vi "main 0.9.1.vi"() -> ()   [LabVIEW 2020]
uses:
  subvi/Newport ESP301/Newport ESP301.lvlib
  subvi/sp_manip.llb/sp_manip_lib.lvlib
  subvi/sp_manip.llb/tcp_gateway.lvlib
  subvi/PHOIBOS/DEFINITIONS/DEF_dev_type.ctl
  subvi/PHOIBOS/DEFINITIONS/DEF_dev_state.ctl
  <vilib>/Utility/file.llb/Write Delimited Spreadsheet (DBL).vi
  <vilib>/Utility/file.llb/Read Delimited Spreadsheet (string).vi
  <vilib>/Analysis/NI_AALBase.lvlib
  <vilib>/Analysis/1siggen.llb/Ramp Pattern by Samples.vi
panel:
  out "Waveform Chart":dbl(graph)
  out "G2 X":cluster{dbl[], "Ramp Pattern":dbl[]}(graph)={array[344 elements], "Ramp Pattern"=[5593.0, 5541.0, 5578.0, 5573.0, 5542.0, 5582.0, 5523.0, 5570.0, 5578.0, 5560.0, 5581.0, 5542.0, 5577.0, 5517.0, 5599.0, 5558.0, 5549.0, 5571.0, 5527.0, 5574.0, 5565.0, 5561.0, 5570.0, 5531.0, 5576.0, 5531.0, 5576.0, 5554.0, 5523.0, 5573.0, 5536.0, 5555.0, 5539.0, 5549.0, 5543.0, 5541.0, 5581.0, 5523.0, 5548.0, 5528.0, 5558.0, 5565.0, 5537.0, 5556.0, 5521.0, 5538.0, 5549.0, 5532.0, 5562.0, 5512.0, 5555.0, 5549.0, 5536.0, 5542.0, 5511.0, 5567.0, 5526.0, 5549.0, 5545.0, 5543.0, 5562.0, 5518.0, 5561.0, 5490.0, 5542.0, 5522.0, 5529.0, 5542.0, 5521.0, 5556.0, 5511.0, 5541.0, 5534.0, 5512.0, 5569.0, 5525.0, 5547.0, 5507.0, 5533.0, 5533.0, 5501.0, 5555.0, 5497.0, 5517.0, 5526.0, 5519.0, 5565.0, 5503.0, 5548.0, 5496.0, 5544.0, 5523.0, 5534.0, 5533.0, 5501.0, 5529.0, 5494.0, 5523.0, 5526.0, 5519.0, 5539.0, 5493.0, 5508.0, 5532.0, 5504.0, 5546.0, 5540.0, 5550.0, 5488.0, 5556.0, 5535.0, 5510.0, 5535.0, 5515.0, 5543.0, 5475.0, 5538.0, 5528.0, 5504.0, 5523.0, 5502.0, 5535.0, 5473.0, 5503.0, 5501.0, 5531.0, 5525.0, 5490.0, 5524.0, 5484.0, 5520.0, 5506.0, 5492.0, 5516.0, 5477.0, 5511.0, 5487.0, 5509.0, 5496.0, 5467.0, 5538.0, 5494.0, 5512.0, 5497.0, 5498.0, 5526.0, 5482.0, 5506.0, 5466.0, 5522.0, 5489.0, 5512.0, 5518.0, 5475.0, 5547.0, 5480.0, 5569.0, 5504.0, 5485.0, 5528.0, 5506.0, 5529.0, 5468.0, 5524.0, 5507.0, 5518.0, 5511.0, 5471.0, 5525.0, 5480.0, 5482.0, 5510.0, 5506.0, 5522.0, 5475.0, 5540.0, 5477.0, 5511.0, 5514.0, 5500.0, 5497.0, 5484.0, 5536.0, 5476.0, 5485.0, 5527.0, 5509.0, 5529.0, 5495.0, 5504.0, 5496.0, 5519.0, 5512.0, 5469.0, 5506.0, 5465.0, 5502.0, 5481.0, 5508.0, 5519.0, 5499.0, 5515.0, 5476.0, 5496.0, 5502.0, 5499.0, 5494.0, 5477.0, 5541.0, 5477.0, 5512.0, 5497.0, 5472.0, 5511.0, 5471.0, 5503.0, 5507.0, 5504.0, 5477.0, 5479.0, 5508.0, 5481.0, 5522.0, 5517.0, 5516.0, 5505.0, 5502.0, 5491.0, 5481.0, 5512.0, 5484.0, 5500.0, 5478.0, 5493.0, 5529.0, 5492.0, 5518.0, 5471.0, 5518.0, 5490.0, 5513.0, 5497.0, 5488.0, 5517.0, 5477.0, 5524.0, 5464.0, 5495.0, 5514.0, 5495.0, 5522.0, 5477.0, 5490.0, 5535.0, 5489.0, 5491.0, 5491.0, 5515.0, 5473.0, 5504.0, 5505.0, 5515.0, 5510.0, 5473.0, 5521.0, 5475.0, 5537.0, 5499.0, 5505.0, 5509.0, 5460.0, 5509.0, 5473.0, 5489.0, 5500.0, 5464.0, 5522.0, 5471.0, 5528.0, 5475.0, 5502.0, 5494.0, 5511.0, 5516.0, 5486.0, 5528.0, 5471.0, 5492.0, 5477.0, 5491.0, 5531.0, 5486.0, 5549.0, 5498.0, 5524.0, 5482.0, 5495.0, 5505.0, 5476.0, 5512.0, 5444.0, 5512.0, 5498.0, 5471.0, 5489.0, 5462.0, 5502.0, 5459.0, 5503.0, 5489.0, 5493.0, 5498.0, 5461.0, 5505.0, 5495.0, 5503.0, 5459.0, 5501.0, 5515.0, 5459.0, 5510.0, 5469.0, 5504.0, 5499.0, 5505.0, 5524.0, 5477.0, 5527.0, 5477.0, 5475.0, 5495.0, 5482.0, 5514.0, 5481.0, 5499.0, 5481.0, 5482.0, 5498.0, 5460.0, 5469.0, 5471.0, 5519.0, 5495.0, 5485.0]}
  in  "reset every n pics":bool
  in  "pics2avg":i32=50
  in  "abort acq.":bool
  out "G2 Y":cluster{dbl[], "Ramp Pattern":dbl[]}(graph)={[5738.0, 5692.0, 5562.0, 5630.0, 5633.0, 5616.0, 5523.0, 5622.0, 5406.0, 5598.0, 5416.0, 5403.0, 5579.0, 5325.0, 5504.0, 5402.0, 5538.0, 5568.0, 5460.0, 5494.0, 5367.0, 5597.0, 5434.0, 5448.0, 5339.0, 5434.0, 5460.0, 5482.0, 5646.0, 5720.0, 5704.0, 5628.0, 5672.0, 5511.0, 5420.0, 5539.0, 5543.0, 5421.0, 5486.0, 5508.0, 5537.0, 5586.0, 5460.0, 5547.0, 5433.0, 5488.0, 5552.0, 5538.0, 5528.0, 5482.0, 5406.0, 5458.0, 5644.0, 5485.0, 5443.0, 5485.0, 5385.0, 5413.0, 5472.0, 5571.0, 5640.0, 5602.0, 5462.0, 5477.0, 5408.0, 5396.0, 5445.0, 5638.0, 5383.0, 5571.0, 5372.0, 5519.0, 5426.0, 5462.0, 5481.0, 5626.0, 5326.0, 5458.0, 5471.0, 5366.0, 5394.0, 5363.0, 5551.0, 5596.0, 5452.0, 5470.0, 5600.0, 5533.0, 5573.0, 5544.0, 5671.0, 5595.0, 5423.0, 5550.0, 5557.0, 5416.0, 5404.0, 5478.0, 5448.0, 5512.0, 5505.0, 5575.0, 5434.0, 5436.0, 5600.0, 5487.0, 5607.0, 5463.0, 5606.0, 5540.0, 5521.0, 5581.0, 5472.0, 5555.0, 5576.0, 5612.0, 5529.0, 5473.0, 5454.0, 5455.0, 5500.0, 5650.0, 5451.0, 5445.0, 5423.0, 5376.0, 5389.0, 5491.0, 5536.0, 5525.0, 5440.0, 5707.0, 5414.0, 5532.0, 5400.0, 5668.0, 5706.0, 5515.0, 5431.0, 5400.0, 5439.0, 5471.0, 5627.0, 5691.0, 5569.0, 5718.0, 5614.0, 5523.0, 5436.0, 5432.0, 5419.0, 5516.0, 5469.0, 5467.0, 5530.0, 5598.0, 5501.0, 5476.0, 5457.0, 5460.0, 5606.0, 5456.0, 5429.0, 5586.0, 5504.0, 5546.0, 5516.0, 5466.0, 5650.0, 5593.0, 5605.0, 5515.0, 5414.0, 5623.0, 5581.0, 5651.0, 5574.0, 5519.0, 5672.0, 5621.0, 5496.0, 5382.0, 5496.0, 5620.0, 5542.0, 5422.0, 5492.0, 5515.0, 5549.0, 5402.0, 5472.0, 5547.0, 5515.0, 5641.0, 5451.0, 5667.0, 5622.0, 5511.0, 5506.0, 5608.0, 5647.0, 5584.0, 5714.0, 5490.0, 5534.0, 5463.0, 5566.0, 5573.0, 5570.0, 5582.0, 5613.0, 5504.0, 5550.0, 5594.0, 5576.0, 5677.0, 5675.0, 5681.0, 5681.0, 5434.0, 5434.0, 5405.0, 5473.0, 5522.0, 5427.0, 5533.0, 5582.0, 5427.0, 5529.0, 5548.0, 5341.0, 5521.0, 5539.0, 5435.0, 5457.0, 5511.0, 5406.0, 5412.0, 5620.0, 5609.0, 5609.0, 5469.0, 5577.0, 5661.0, 5673.0, 5518.0, 5463.0, 5562.0, 5723.0, 5719.0, 5487.0, 5485.0, 5683.0, 5501.0, 5604.0, 5328.0], "Ramp Pattern"=[0.0, 1.003921568627451, 2.007843137254902, 3.011764705882353, 4.015686274509804, 5.019607843137255, 6.023529411764706, 7.027450980392157, 8.031372549019608, 9.035294117647059, 10.03921568627451, 11.04313725490196, 12.047058823529412, 13.050980392156863, 14.054901960784314, 15.058823529411764, 16.062745098039215, 17.066666666666666, 18.070588235294117, 19.07450980392157, 20.07843137254902, 21.08235294117647, 22.08627450980392, 23.090196078431372, 24.094117647058823, 25.098039215686274, 26.101960784313725, 27.105882352941176, 28.109803921568627, 29.113725490196078, 30.11764705882353, 31.12156862745098, 32.12549019607843, 33.129411764705885, 34.13333333333333, 35.13725490196079, 36.141176470588235, 37.14509803921569, 38.14901960784314, 39.15294117647059, 40.15686274509804, 41.16078431372549, 42.16470588235294, 43.168627450980395, 44.17254901960784, 45.1764705882353, 46.180392156862744, 47.1843137254902, 48.188235294117646, 49.1921568627451, 50.19607843137255, 51.2, 52.20392156862745, 53.207843137254905, 54.21176470588235, 55.21568627450981, 56.219607843137254, 57.22352941176471, 58.227450980392156, 59.23137254901961, 60.23529411764706, 61.23921568627451, 62.24313725490196, 63.247058823529414, 64.25098039215686, 65.25490196078431, 66.25882352941177, 67.26274509803922, 68.26666666666667, 69.27058823529411, 70.27450980392157, 71.27843137254902, 72.28235294117647, 73.28627450980392, 74.29019607843138, 75.29411764705883, 76.29803921568627, 77.30196078431372, 78.30588235294118, 79.30980392156863, 80.31372549019608, 81.31764705882352, 82.32156862745099, 83.32549019607843, 84.32941176470588, 85.33333333333333, 86.33725490196079, 87.34117647058824, 88.34509803921569, 89.34901960784313, 90.3529411764706, 91.35686274509804, 92.36078431372549, 93.36470588235294, 94.3686274509804, 95.37254901960785, 96.37647058823529, 97.38039215686274, 98.3843137254902, 99.38823529411765, 100.3921568627451, 101.39607843137254, 102.4, 103.40392156862745, 104.4078431372549, 105.41176470588235, 106.41568627450981, 107.41960784313726, 108.4235294117647, 109.42745098039215, 110.43137254901961, 111.43529411764706, 112.43921568627451, 113.44313725490196, 114.44705882352942, 115.45098039215686, 116.45490196078431, 117.45882352941176, 118.46274509803922, 119.46666666666667, 120.47058823529412, 121.47450980392156, 122.47843137254903, 123.48235294117647, 124.48627450980392, 125.49019607843137, 126.49411764705883, 127.49803921568628, 128.50196078431372, 129.50588235294117, 130.50980392156862, 131.51372549019607, 132.51764705882354, 133.521568627451, 134.52549019607844, 135.52941176470588, 136.53333333333333, 137.53725490196078, 138.54117647058823, 139.54509803921567, 140.54901960784315, 141.5529411764706, 142.55686274509804, 143.5607843137255, 144.56470588235294, 145.5686274509804, 146.57254901960783, 147.57647058823528, 148.58039215686276, 149.5843137254902, 150.58823529411765, 151.5921568627451, 152.59607843137255, 153.6, 154.60392156862744, 155.6078431372549, 156.61176470588236, 157.6156862745098, 158.61960784313726, 159.6235294117647, 160.62745098039215, 161.6313725490196, 162.63529411764705, 163.6392156862745, 164.64313725490197, 165.64705882352942, 166.65098039215687, 167.65490196078431, 168.65882352941176, 169.6627450980392, 170.66666666666666, 171.6705882352941, 172.67450980392158, 173.67843137254903, 174.68235294117648, 175.68627450980392, 176.69019607843137, 177.69411764705882, 178.69803921568626, 179.7019607843137, 180.7058823529412, 181.70980392156864, 182.71372549019608, 183.71764705882353, 184.72156862745098, 185.72549019607843, 186.72941176470587, 187.73333333333332, 188.7372549019608, 189.74117647058824, 190.7450980392157, 191.74901960784314, 192.75294117647059, 193.75686274509803, 194.76078431372548, 195.76470588235293, 196.7686274509804, 197.77254901960785, 198.7764705882353, 199.78039215686275, 200.7843137254902, 201.78823529411764, 202.7921568627451, 203.79607843137254, 204.8, 205.80392156862746, 206.8078431372549, 207.81176470588235, 208.8156862745098, 209.81960784313725, 210.8235294117647, 211.82745098039214, 212.83137254901962, 213.83529411764707, 214.8392156862745, 215.84313725490196, 216.8470588235294, 217.85098039215686, 218.8549019607843, 219.85882352941175, 220.86274509803923, 221.86666666666667, 222.87058823529412, 223.87450980392157, 224.87843137254902, 225.88235294117646, 226.8862745098039, 227.89019607843136, 228.89411764705883, 229.89803921568628, 230.90196078431373, 231.90588235294118, 232.90980392156862, 233.91372549019607, 234.91764705882352, 235.92156862745097, 236.92549019607844, 237.9294117647059, 238.93333333333334, 239.93725490196078, 240.94117647058823, 241.94509803921568, 242.94901960784313, 243.95294117647057, 244.95686274509805, 245.9607843137255, 246.96470588235294, 247.9686274509804, 248.97254901960784, 249.9764705882353, 250.98039215686273, 251.98431372549018, 252.98823529411766, 253.9921568627451, 254.99607843137255, 256.0]}
  out "ETA":timestamp=timestamp(3543843884.995538 s since 1904-01-01) format="%<%H:%M:%S>T"
  out "acq. imgs":i32=30
  out "snap_prog":dbl(slide)=1.0 scale=0.0..1.0
  in  "BasePath":path=path "Z:/PESdata"
  in  "cam_liveavg":bool caption="live average"
  out "cam_fps":dbl=20.079713544692744 caption="FPS" format="%.1g"
  out "sideimg":dbl[][](graph)
  in  "RunNumber":u16=77
  out "sum":dbl=4126991.0 format="%#.2g"
  out "max":dbl=54.0
  out "mainimg":dbl[][](graph)
  out "ESP_con?":bool=TRUE caption="ESP301"
  out "phoib_con?":bool caption="PHOIBOS"
  out "manip_con?":bool caption="manipulator"
  out "cam_con?":bool caption="camera"
  in  "main_close":bool
  in  "Tab Control":T1(tab)
  in  "manip_deltas":dbl[](array[numeric])=[0.0, 0.0, 0.0, 0.0, 10.0, 0.0] caption="delta" format="%#.5g"
  in  "aq.mode":enum32{"Radio Selection 1", "Radio Selection 2"}(radio)=enum."Radio Selection 2"
  in  "dark avg":i32=100
  in  "averages":i32=30 caption="N"
  in  "ESP_delta":dbl caption="relative [mm]"
  in  "ESP_-":bool
  in  "ESP_+":bool
  in  "ESP_go":bool
  in  "ESP_dest_t":dbl=250.17307139859977 caption="[fs]"
  in  "ESP_dest":dbl=31.304 caption="[mm]"
  in  "ESP_set_t0":bool
  in  "phoib_I_6s":dbl=3200.0
  in  "phoib_I_5s":dbl=1650.0
  in  "phoib_I_4s":dbl=4.558
  in  "phoib_I_3s":dbl=-7.0
  in  "phoib_I_2s":dbl=20.0
  in  "phoib_I_1s":dbl=22.0
  in  "phoib_standby":bool
  in  "phoib_set":bool
  out "phoib_I_6":dbl caption="Screen Voltage"
  out "phoib_I_5":dbl caption="Detctor Voltage"
  out "phoib_I_4":dbl caption="Work Function"
  out "phoib_I_3":dbl caption="Coil Current"
  out "phoib_I_2":dbl caption="Pass Energy"
  out "phoib_I_1":dbl caption="Kinetic Energy"
  out "Saved Positions":string[][](table)=[["ertwertwert", "-2.299945", "-2.030214", "38.900024", "50.000762", "0.000887", "-97.998082"], ["uztgugt", "-14.999451", "-13.638894", "442.380066", "13.998380", "-1.893758", "-76.305838"], ["asdf", "-14.999451", "-13.638894", "442.380066", "13.998380", "-1.893758", "-76.305838"], ["test3", "-14.999451", "-13.638894", "441.380066", "13.998380", "-1.893758", "-76.305838"]]
  in  "Save Pos":bool
  in  "Load":bool
  in  "Delete":bool
  in  "ManipRel +":bool
  in  "ManipRel -":bool
  in  "Move Abs":bool
  in  "stop manip":bool
  in  "dest":dbl[](array[numeric])=[-2.6172862113166087, -0.009888298846365134, 68.5008544921875, -46.36280498847848, 1.1073518432055398, -218.56360350415366] caption="destination" format="%#.5g"
  out "axis":string[](array[string])=["x", "y", "z", "polar", "tilt", "azimut"]
  out "pos":dbl[](array[numeric])=[-2.6172862113166087, -0.009888298846365134, 68.5008544921875, -46.363686276590336, 11.108982061941884, -218.56360350415366] caption="position" format="%.5f"
  in  "Mode":T2(ring)=enum."WideAngleMode"
  in  "VoltageRange":enum16{"3.5kV", "1.5kV", "400V", "100V", "10V"}(ring)=enum."400V"
  out "ESP_pos":dbl=31.4539 caption="Position"
  out "ESP_delay":dbl=1000.0251574040756 caption="Delay"
  out "ESP_t0":dbl=31.304 caption="Time Zero @"
  out "phoib_I_7":dbl caption="Conversion Voltage"
  in  "phoib_I_7s":dbl=-16.0
  in  "phoib_I_8s":dbl=0.0039
  in  "phoib_I_9s":dbl=0.0039
  out "phoib_I_8":dbl caption="FD1"
  out "phoib_I_9":dbl caption="FD2"
  in  "gain":bool
  in  "exposure [ms]":u32=1
  in  "binning":u16(ring)=2 items=["X 1", "X 2", "X 4", "X 8"]
  in  "cam_dark?":bool caption="subtract dark?"
  in  "cam_dark":bool
  in  "cam_saveimg":bool
  in  "e-size":u8
  in  "lower threshold":i32=-100
  in  "count?":bool
  in  "ROI Left":i32=1
  in  "ROI Right":i32=43
  in  "ROI Top":i32=1
  in  "ROI Bottom":i32=33
  out "moving?":bool[](array[boolean])
  out "del_ETA":timestamp=timestamp(3543843871.185777 s since 1904-01-01) format="%<%H:%M:%S>T"
  out "time / step":dbl=2.792118032773336
  out "duration [HH:MM:SS]":dbl=55.62603882380894 format="%<%H:%M:%S>t"
  out "disk [MB]":dbl=11.613000000000001
  out "RAM [MB]":dbl=2.765
  out "total steps":dbl=20.0
  out "delaypoints":dbl=5.0
  in  "generate delay table":bool
  in  "load delay table":bool
  in  "delay table [fs]":string[][](table)=[["-1000.000000"], ["-500.000000"], ["0.000000"], ["500.000000"], ["1000.000000"]]
  in  "delscan_iters":u32=4 caption="iterations"
  out "scangraph":cluster{"delaypoints":dbl[], dbl[]}(graph)={"delaypoints"=[-1000.0, -500.0, 0.0, 500.0, 1000.0], [56872639.0, 56944859.59999999, 56835838.7999999, 56879783.599999934, 56864774.39999998]}
  in  "delscan_abort":bool
  out "delscan_progress":u32(slide)=5 scale=0.0..5.0
  in  "delscan_go":bool
  out "delscan_pos":dbl=31.453896228999998 caption="stage pos [mm]"
  in  "delscan_end":dbl=1000.0 caption="end [fs]"
  in  "delscan_stepsize":dbl=500.0 caption="stepsize [fs]"
  in  "delscan_start":dbl=-1000.0 caption="start [fs]"
  out "iteration":i32=5
  in  "delscan_finishIteration":bool
  in  "manip_scan_steps":u32=3
  in  "Optimize":bool
  in  "manip_scan_delta":dbl[](array[numeric])=[0.0, 0.0, 0.0, 0.0, 1.0, 0.0] caption="delta" format="%#.5g"
  out "delscan_progress 2":u32(slide)=2 scale=0.0..3.0
  in  "abort":bool
  in  "manip_init":bool
  in  "manip_release":bool
  in  "phoib_init":bool
  in  "phoib_release":bool
  in  "ESP_init":bool
  in  "ESP_release":bool
  in  "ESP301 VISA":refnum<visa-resource-name>="COM8"
  in  "board number":i32
  in  "cam_init":bool
  in  "cam_release":bool
  out "cam_error":errorcluster
  out "phoib_error":errorcluster
  out "state":T3 items=["Off"=-1, "Standby"=0, "On"=1]
  in  "ESP Axis":i32=1 min=1 max=3
  out "error out":errorcluster
  out "error out 2":errorcluster={"status"=TRUE, "code"=1, "source"="TCP Write in sp_manip_lib.lvlib:sp_manip_disconnect.vi->main 0.9.1.vi"}
  # "camera"
  # "analyzer"
  # "manipulator"
  # "aquisition"
  # "delay stage"
  # "Position"
  # "Destination"
  # "X\nY\nZ\npolar\ntilt\nazimut"
  # "camera"
  # "phoibos"
  # "ESP301"
  # "manipulator"
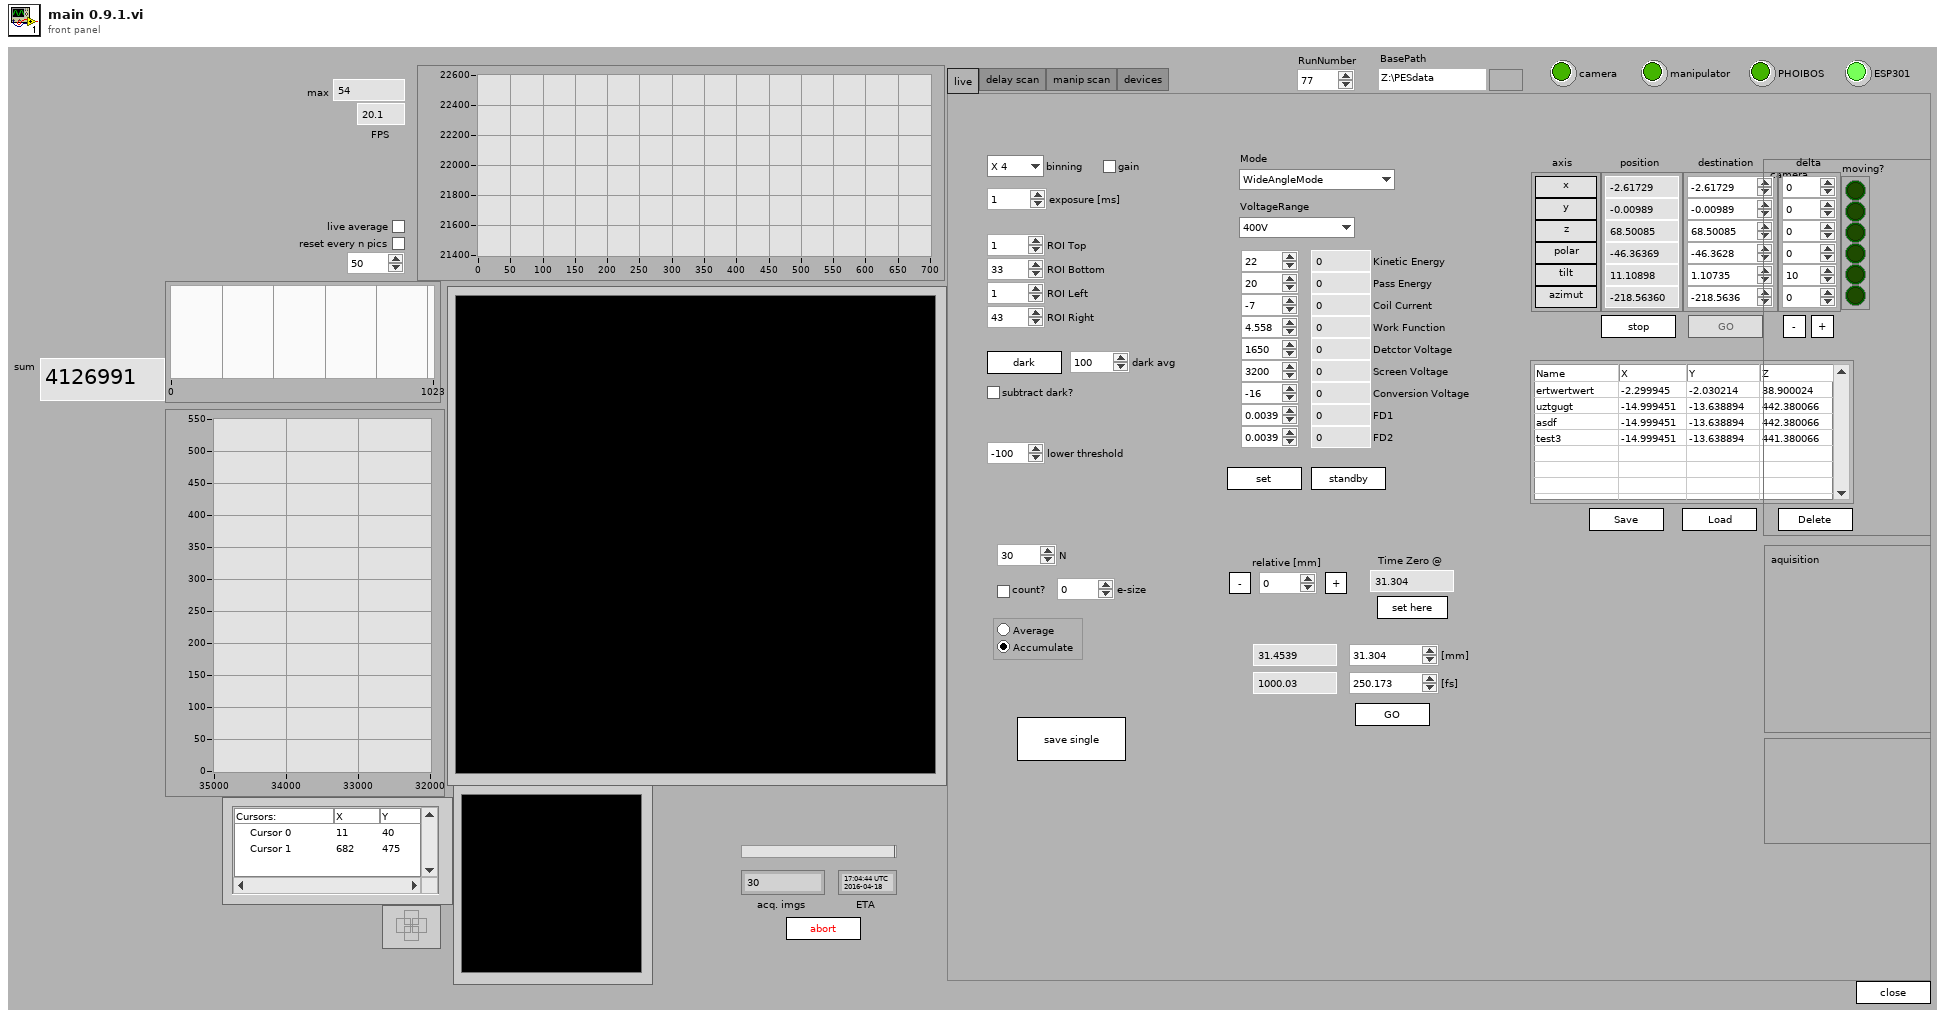
[diagram p1: front panel]
types:
  T1 = enum32{"live", "delay scan", "manip scan", "devices"}
  T2 = enum16{"HighMagnification", "MediumMagnification", "LowMagnification", "HighAngularDispersion", "MediumAngularDispersion", "LowAngularDispersion", "WideAngleMode", "LargeArea", "MediumArea", "SmallArea", "HighMagnification2", "SmallArea2", "ImagingMode"}
  T3 = typedef "DEF_dev_state.ctl" = i32
  T4 = typedef "LVCursorListTypeDef.ctl" = cluster{"Name":string, "Color":u32, "Style":u8, "Point Style":u8, "Name Visible":bool, "Allow Drag":bool, "Cursor Mode":u32, "Plot":i32, "Index":i32, "Position":cluster{"X":dbl, "Y":dbl}, "X Scale":u32, "Y Scale":u32, "Watch Plots":i32[], "Watch All Plots":bool, "Plot Area":i32, "Label Offset":cluster{"X":dbl, "Y":dbl}}[]
  T5 = cluster{"Camera type":u32, "Operating mode\nHP & QE / HS & DiCam Pro ":u32, "Frame trigger \n(High Performance and QE only)":u16, "Sequence trigger":u16, "Low Light\n(QE only)":bool, "Gain":bool, "Horzontal\nbinning":u16, "Vertical\nbinning ":u16, "ROI Left":i32, "ROI Right":i32, "ROI Top":i32, "ROI Bottom":i32}
  T6 = cluster{"Name":string, "Color":u32, "Style":u8, "Point Style":u8, "Name Visible":bool, "Allow Drag":bool, "Cursor Mode":u32, "Plot":i32, "Index":i32, "Position":cluster{"X":dbl, "Y":dbl}, "X Scale":u32, "Y Scale":u32, "Watch Plots":i32[], "Watch All Plots":bool, "Plot Area":i32, "Label Offset":cluster{"X":dbl, "Y":dbl}}
  T7 = cluster{"Axis_Name":string, "Axis_Type":string, "Axis_Position":dbl, "continous":bool, "moving":bool}[]
  T8 = typedef "DEF_dev_type.ctl" = enum32{"devA (analyzer)", "devD (detector)"}
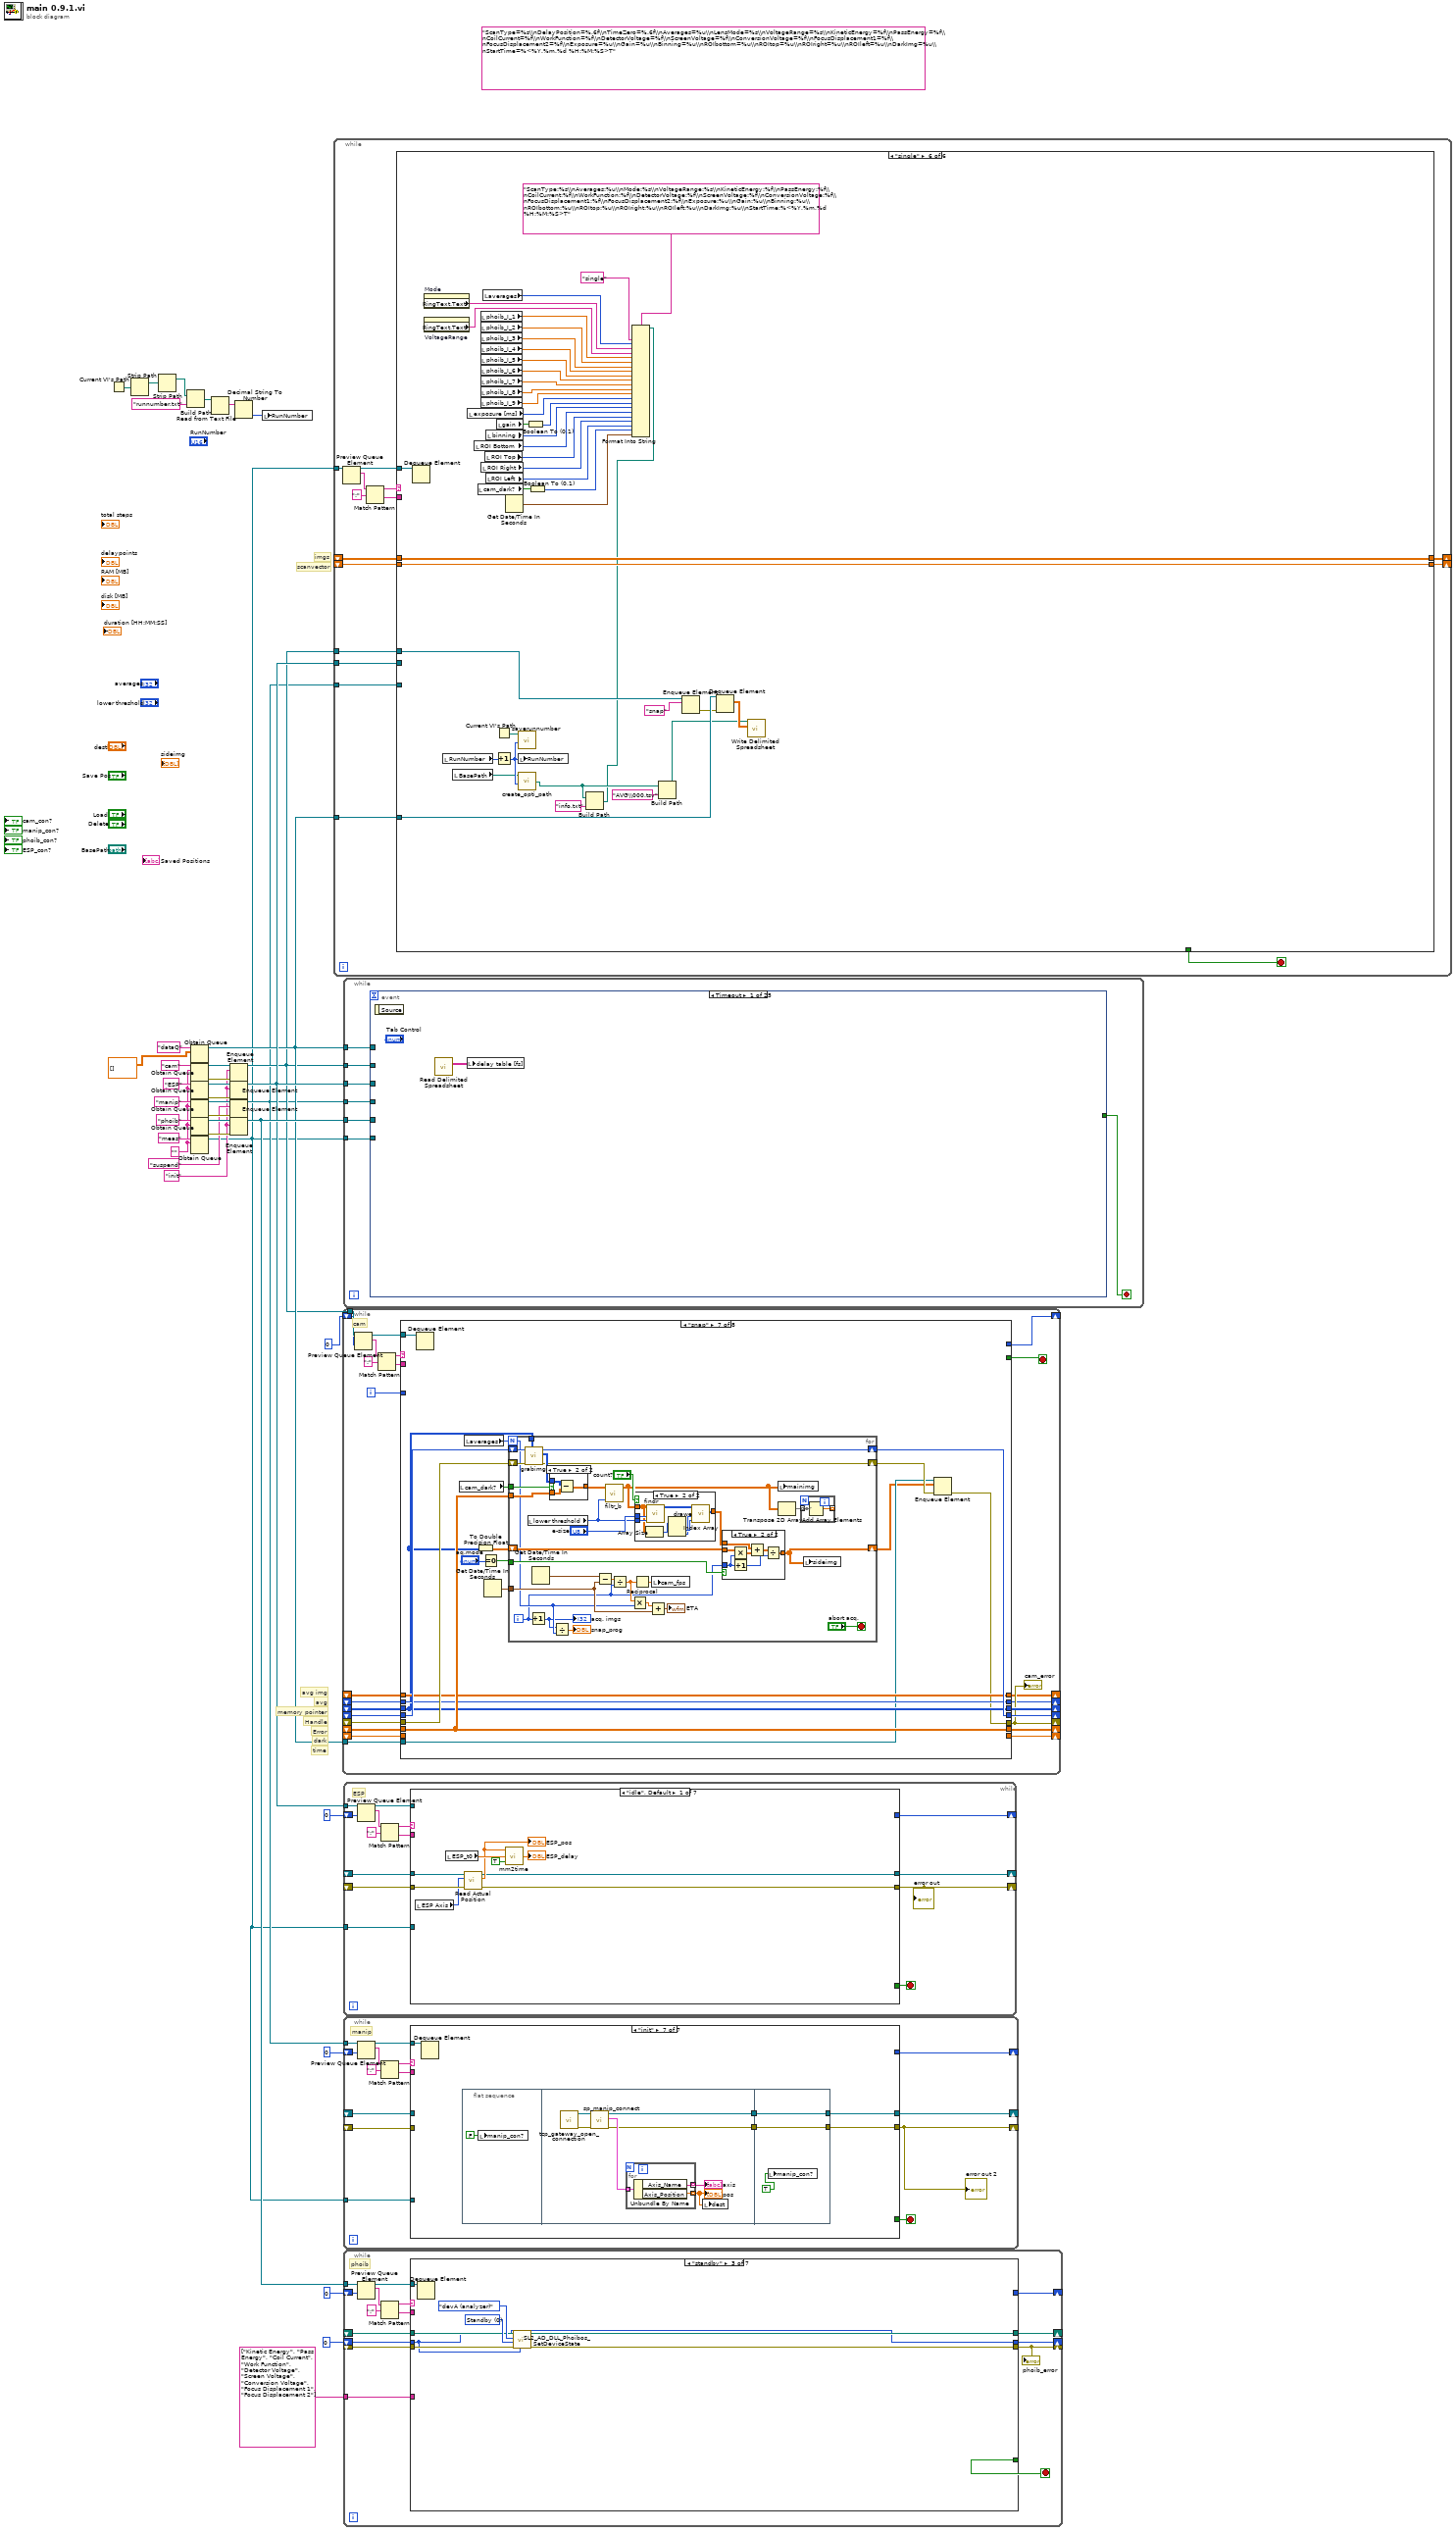
[diagram p0: block diagram]
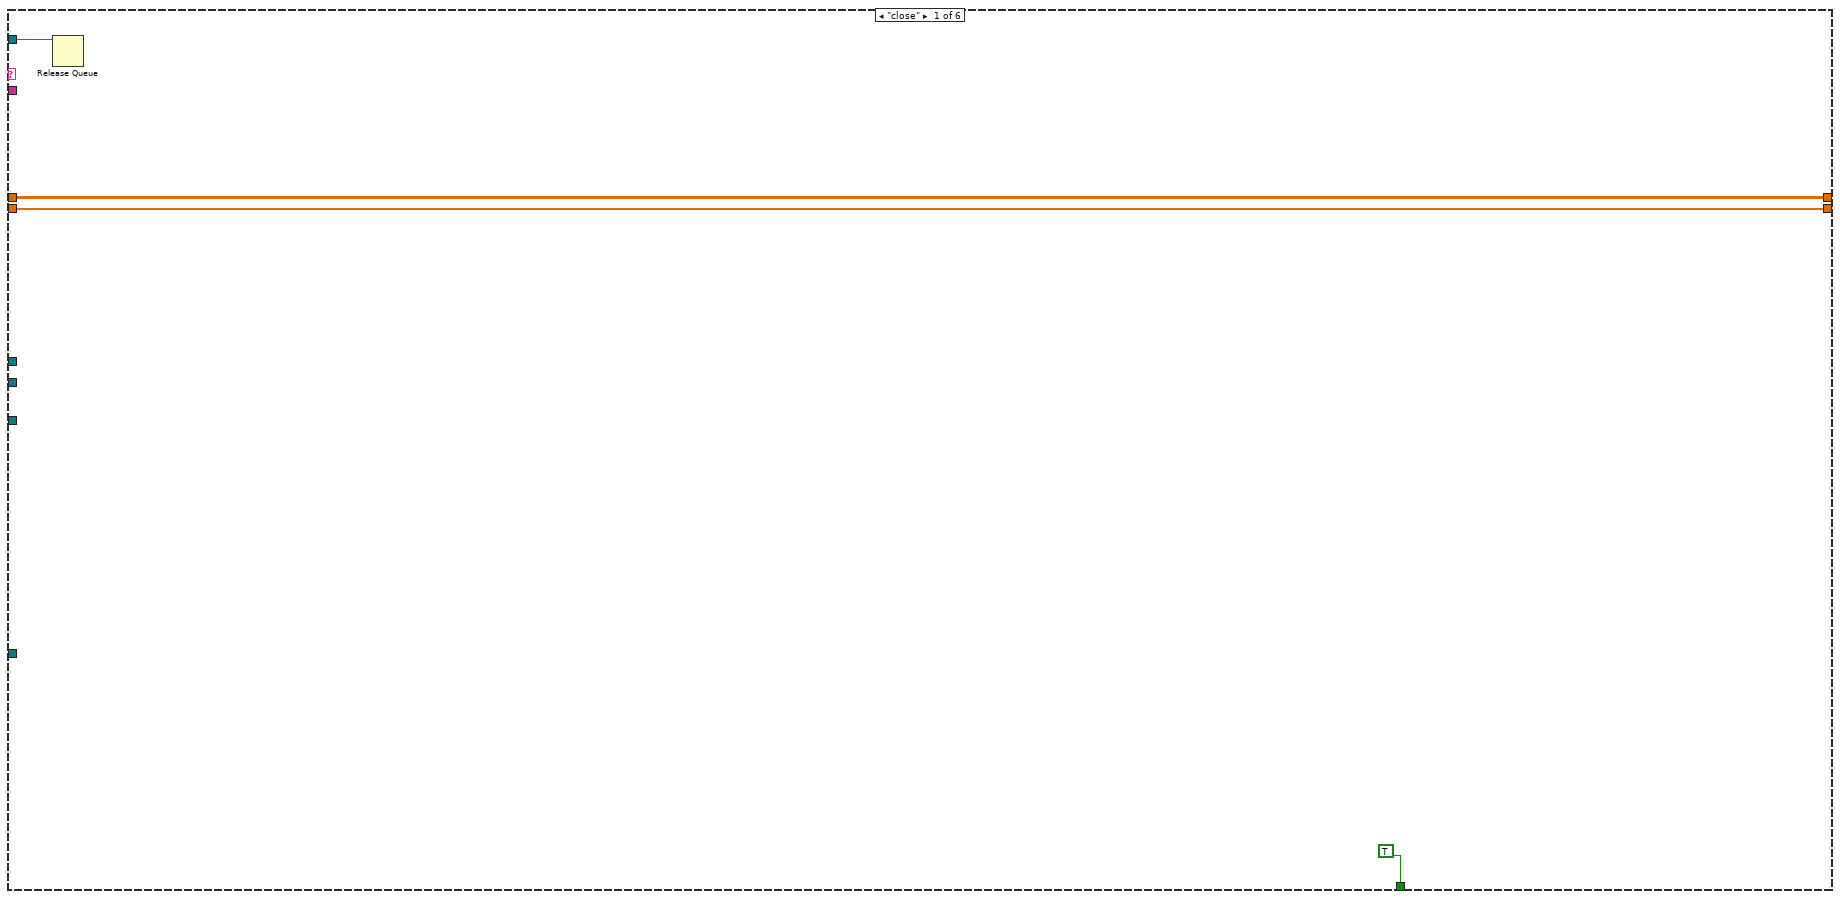
[diagram p2: hidden frame]
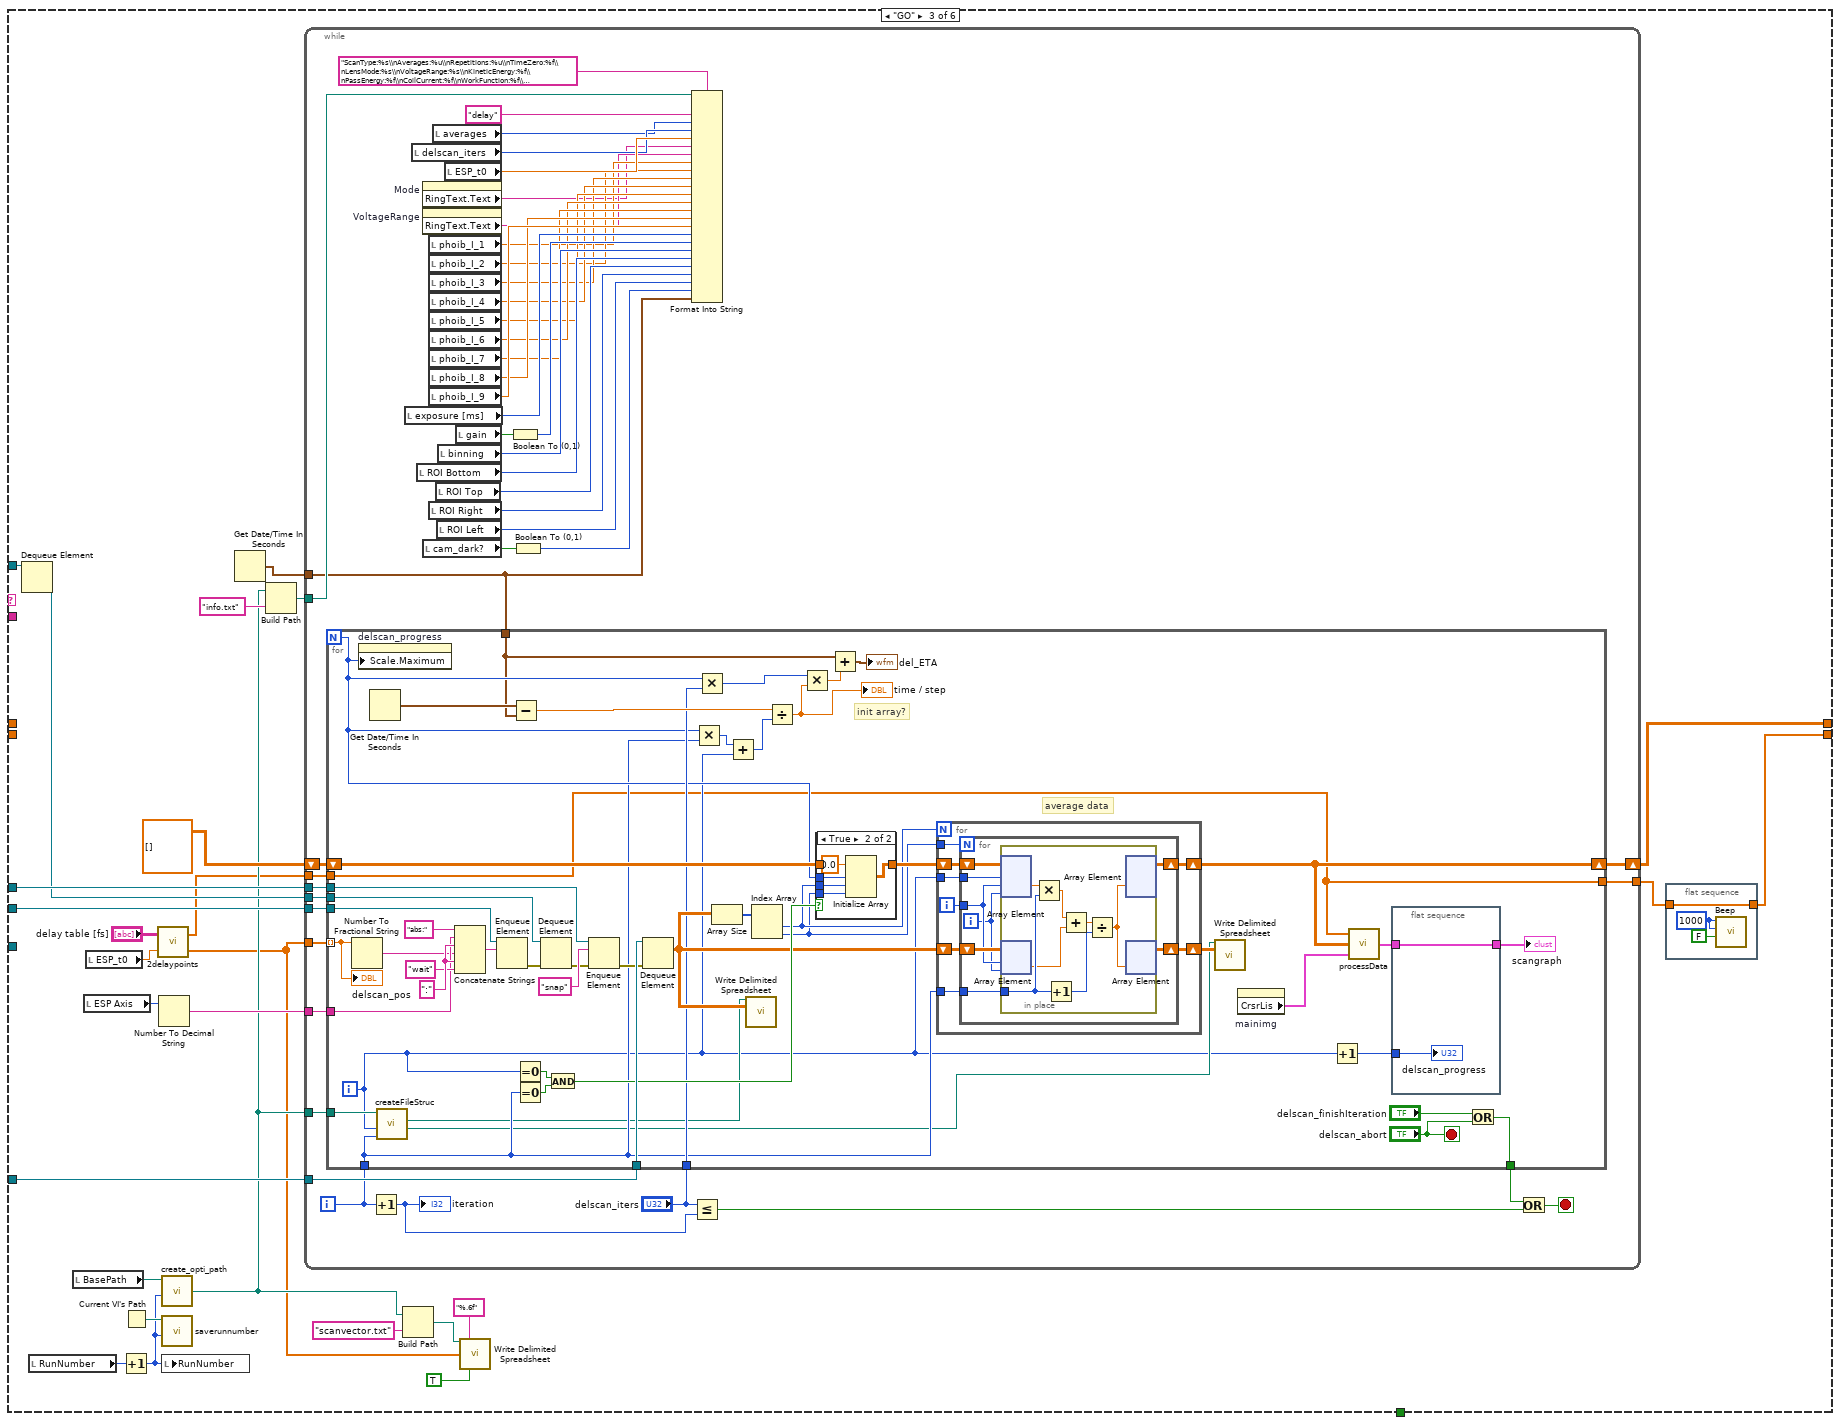
[diagram p4: hidden frame]
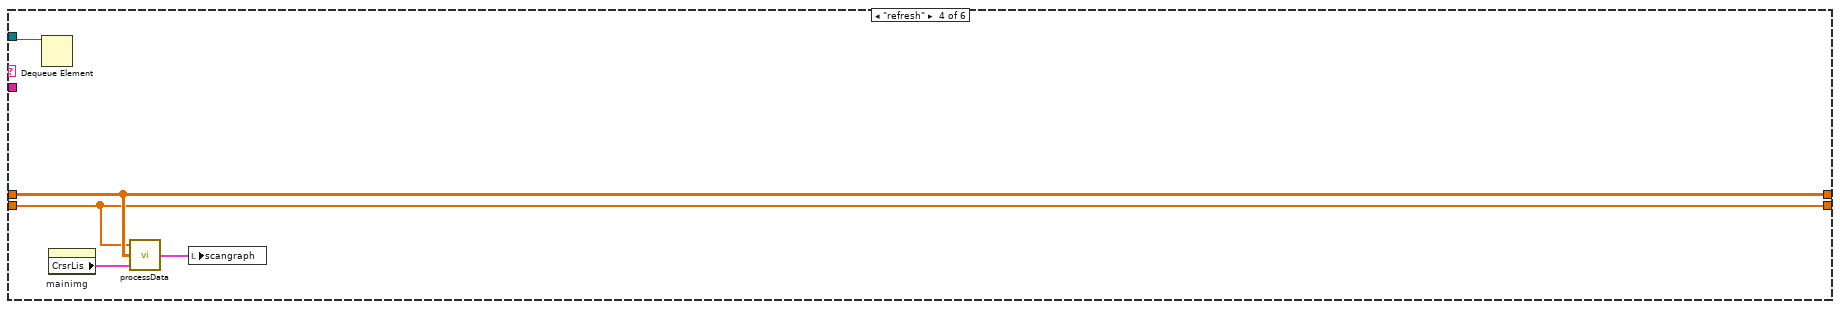
[diagram p6: hidden frame]
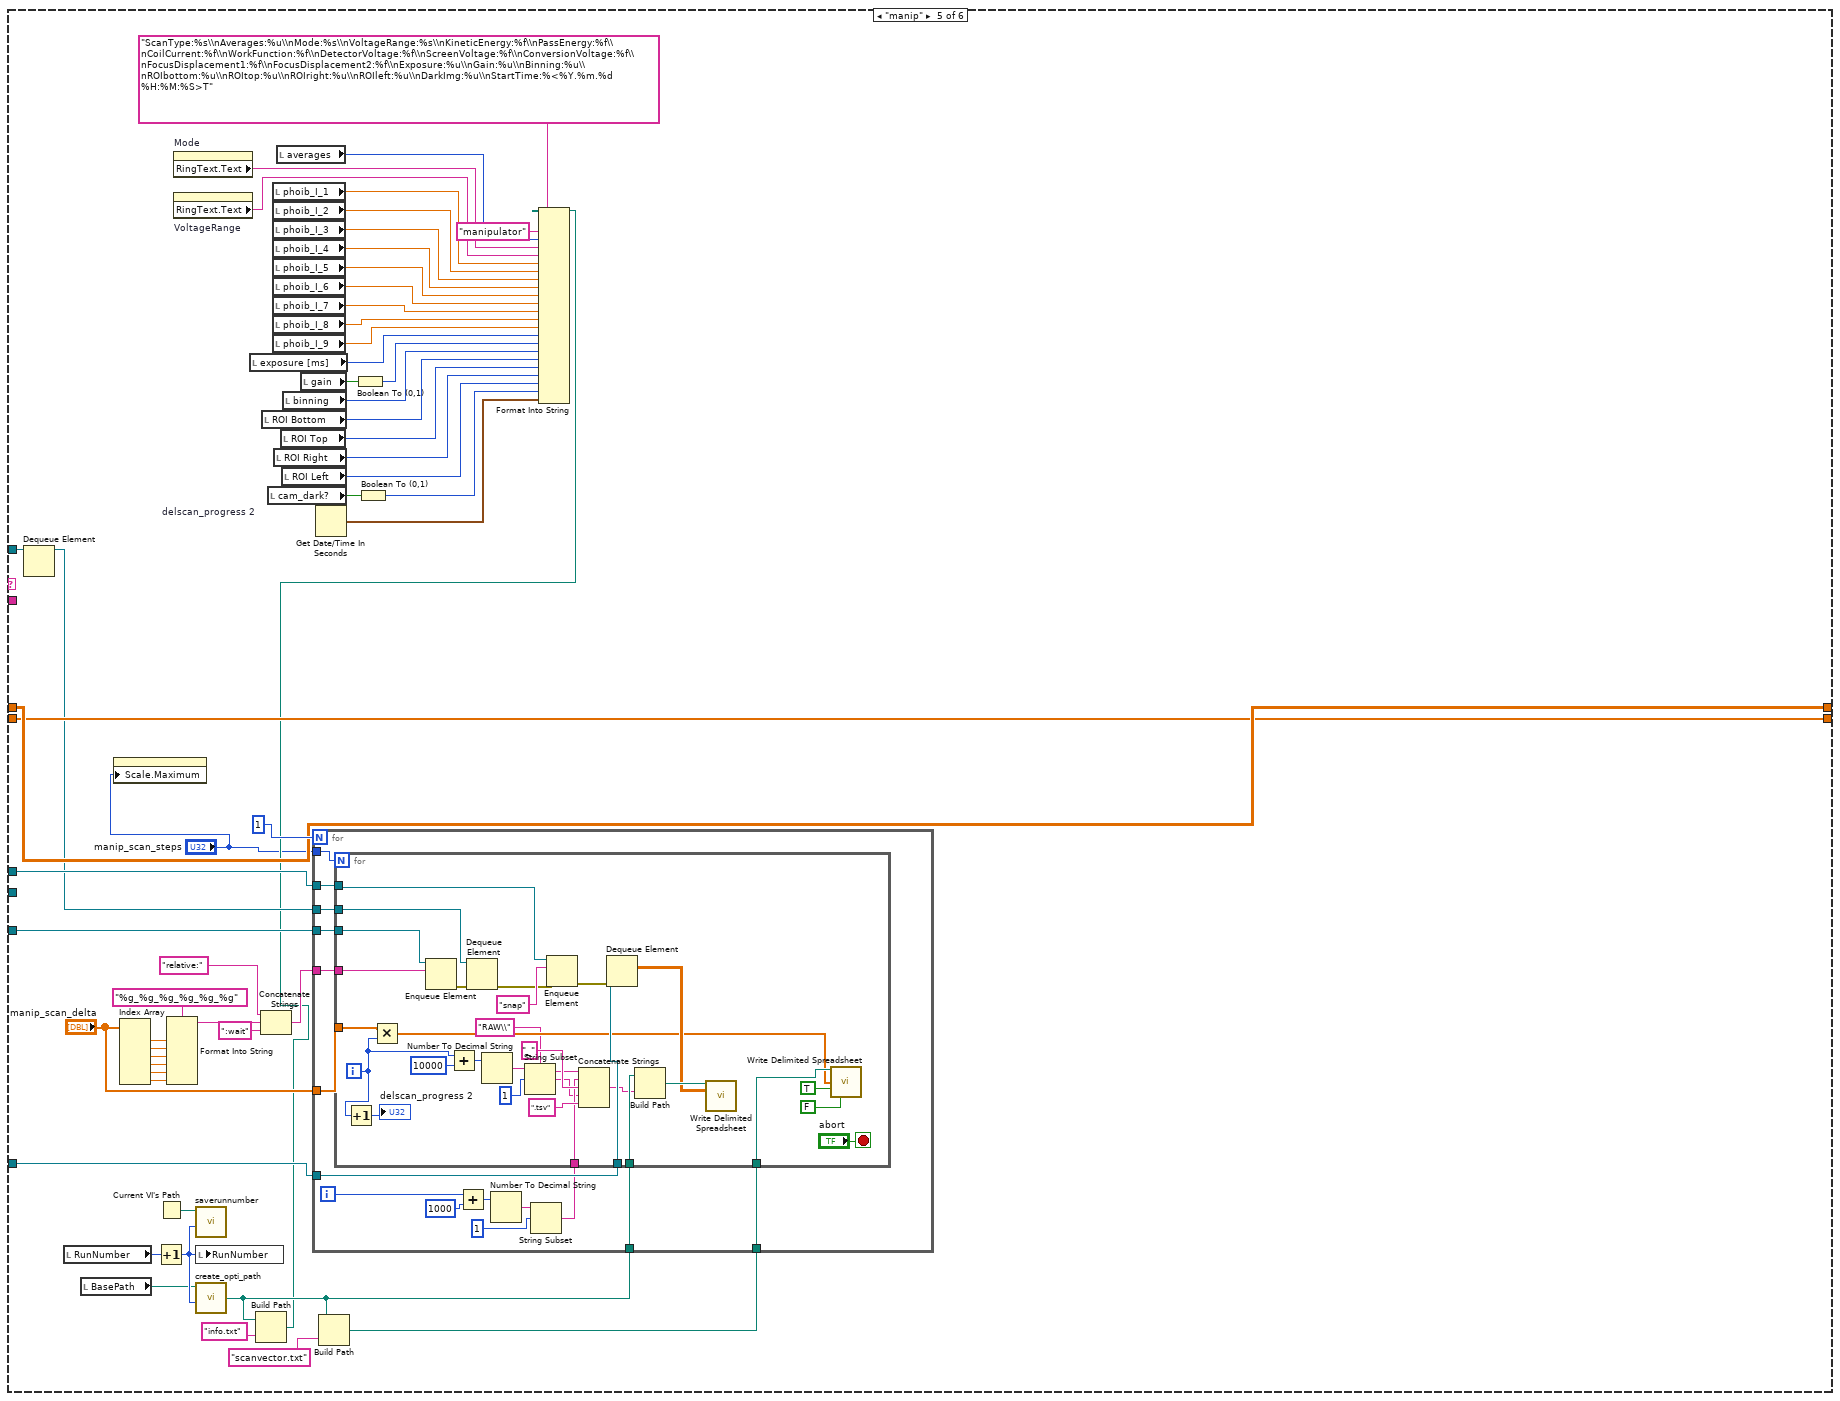
[diagram p7: hidden frame]
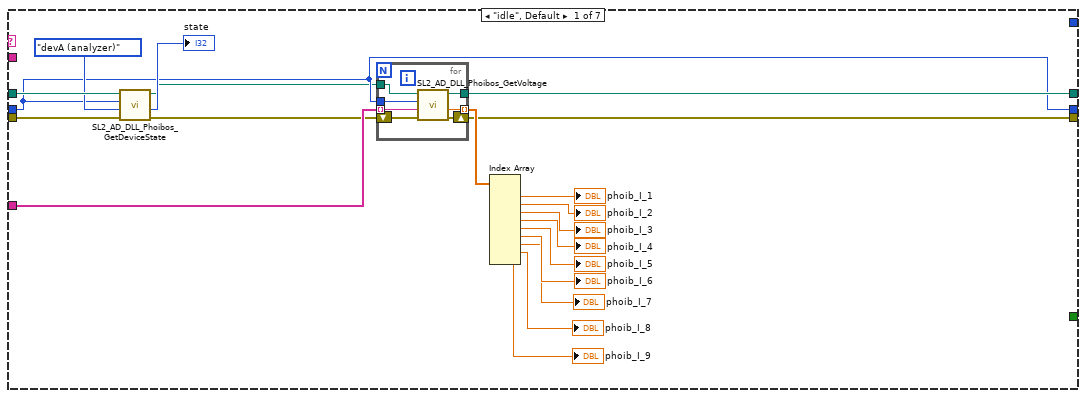
[diagram p8: hidden frame]
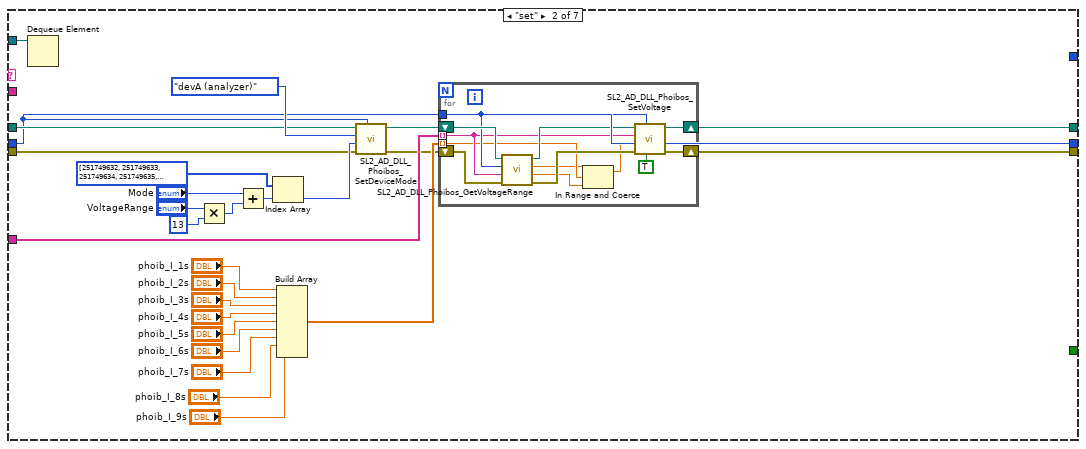
[diagram p9: hidden frame]
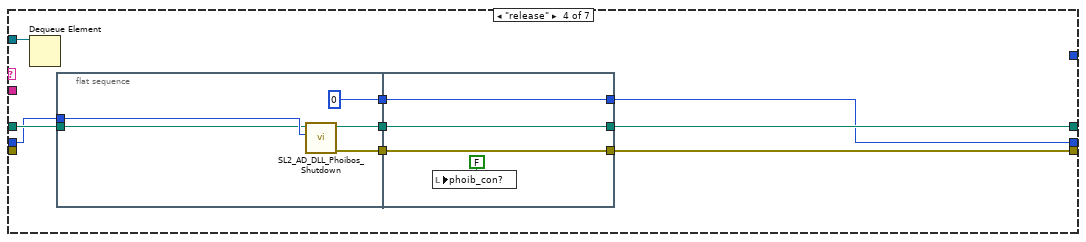
[diagram p10: hidden frame]
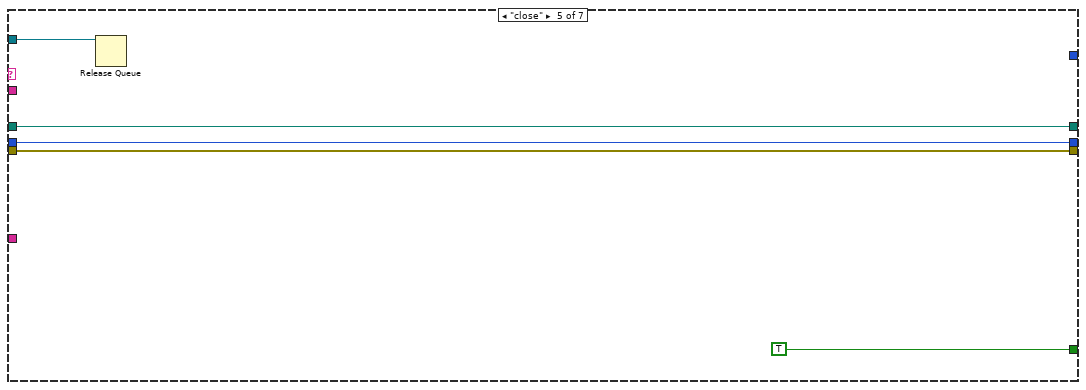
[diagram p11: hidden frame]
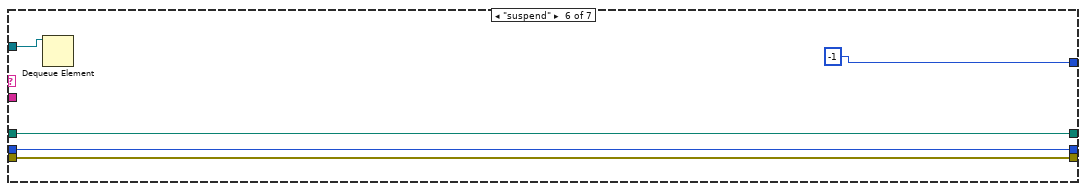
[diagram p12: hidden frame]
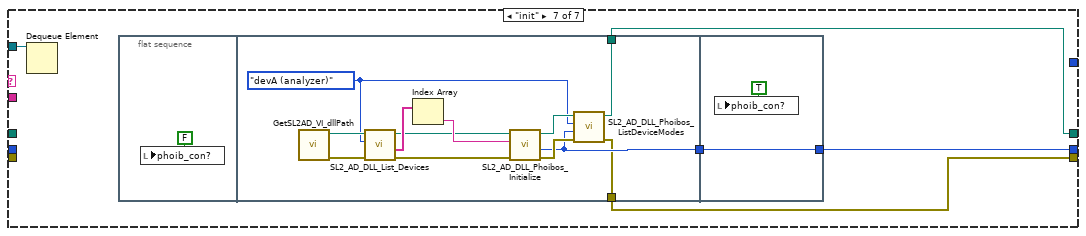
[diagram p13: hidden frame]
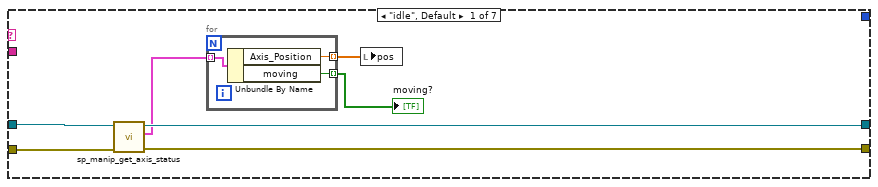
[diagram p14: hidden frame]
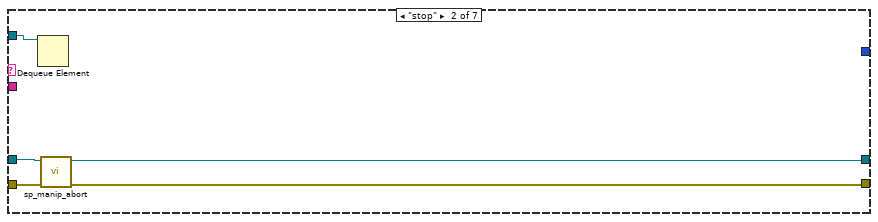
[diagram p15: hidden frame]
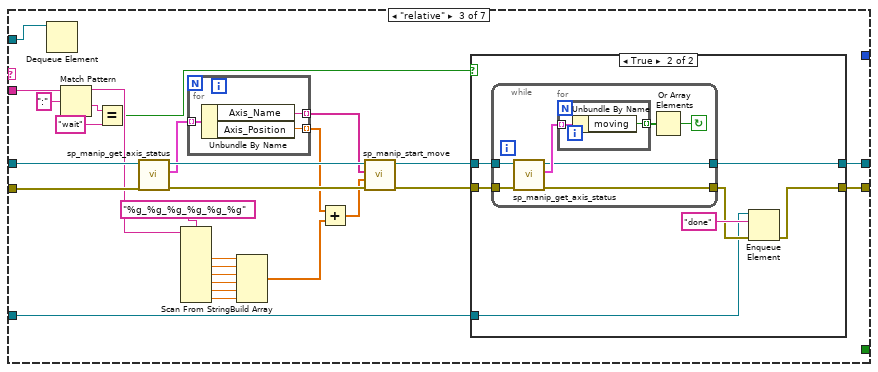
[diagram p16: hidden frame]
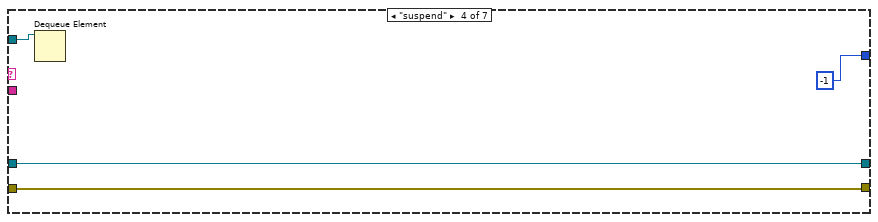
[diagram p18: hidden frame]
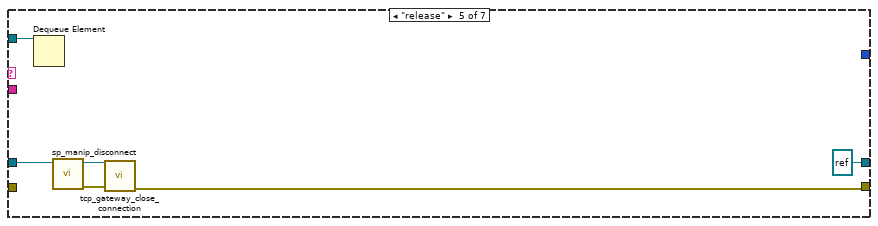
[diagram p19: hidden frame]
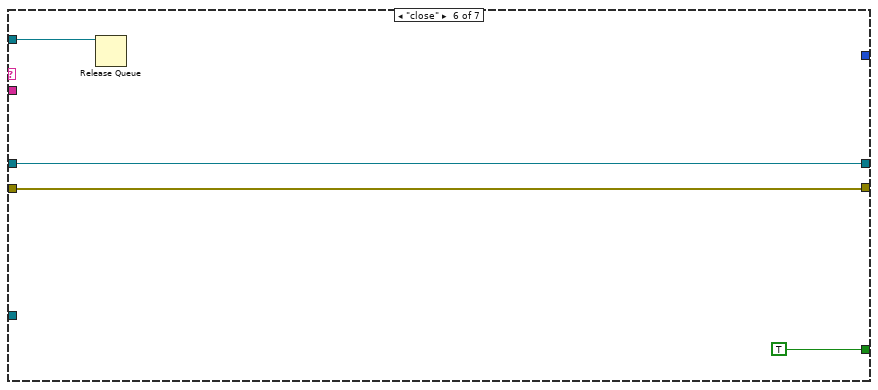
[diagram p20: hidden frame]
diagram:
  (unwired) "ScanType=%s\\nDelayPosition=%.6f\\nTimeZero=%.6f\\nAverages=%u\\nLensMode=%s\\nVoltageRange=%s\\nKineticEnergy=%f\\nPassEnergy=%f\\nCoilCurrent=%f\\nWorkFunction=%f\\nDetectorVoltage=%f\\nScreenVoltage=%f\\nConversionVoltage=%f\\nFocusDisplacement1=%f\\nFocusDisplacement2=%f\\nExposure=%u\\nGain=%u\\nBinning=%u\\nROIbottom=%u\\nROItop=%u\\nROIright=%u\\nROIleft=%u\\nDarkImg=%u\\nStartTime=%<%Y.%m.%d %H:%M:%S>T" ("format string")
  w14 = "init" ("name (unnamed)")
  w16 = "" ("name (unnamed)")
  # "scanvector"
  # "imgs"
  # "avg img"
  # "avg"
  # "time"
  # "dark"
  # "Error"
  # "Handle"
  # "memory pointer"
  n1 = Current VI's Path() -> (path=w4:path)
  n2 = Strip Path(path=w4) -> (stripped path=w8:path)  [unwired: 1 out]
  n3 = Strip Path(path=w8) -> (stripped path=w9:path)  [unwired: 1 out]
  n4 = Build Path(base path=w9, name or relative path="runnumber.txt") -> (appended path=w6:path)
  n5 = Obtain Queue(name (unnamed)="dataQ", element data type=dbl[][] []) -> (queue out=w11:refnum<queue>)  [unwired: 3 in, 2 out]
  n6 = Obtain Queue(name (unnamed)="cam", element data type=w16) -> (queue out=w36:refnum<queue>, error out=w35:errorcluster)  [unwired: 3 in, 1 out]
  n7 = Obtain Queue(name (unnamed)="ESP", element data type=w16) -> (queue out=w33:refnum<queue>, error out=w34:errorcluster)  [unwired: 3 in, 1 out]
  n8 = Obtain Queue(name (unnamed)="manip", element data type=w16) -> (queue out=w30:refnum<queue>, error out=w29:errorcluster)  [unwired: 3 in, 1 out]
  n9 = Obtain Queue(name (unnamed)="phoib", element data type=w16) -> (queue out=w27:refnum<queue>, error out=w28:errorcluster)  [unwired: 3 in, 1 out]
  n10 = Obtain Queue(name (unnamed)="meas", element data type=w16) -> (queue out=w2:refnum<queue>)  [unwired: 3 in, 2 out]
  n11 = Read from Text File(file (use dialog)=w6) -> (text=w7:string)  [unwired: 3 in, 3 out]
  n12 = Enqueue Element(queue=w36, element=w14, error in (no error)=w35) -> (queue out=w10:refnum<queue>)  [unwired: 1 in, 2 out]
  n13 = Enqueue Element(queue=w33, element=w14, error in (no error)=w34) -> (queue out=w13:refnum<queue>)  [unwired: 1 in, 2 out]
  n14 = Enqueue Element(queue=w30, element="suspend" ("name (unnamed)"), error in (no error)=w29) -> (queue out=w3:refnum<queue>)  [unwired: 1 in, 2 out]
  n15 = Enqueue Element(queue=w27, element=w14, error in (no error)=w28) -> (queue out=w24:refnum<queue>)  [unwired: 1 in, 2 out]
  n16 = Decimal String To Number(string=w7) -> (number=w1:i32)  [unwired: 2 in, 1 out]
  n17 = local write "RunNumber"(w1) -> ()
  n18 = while {
    tunnel: w11 -> [w52]
    tunnel: w13 -> [w51]
    tunnel: w10 -> [w50]
    shift-right: [w47] -> _
    shift-left: _ -> [w49]
    shift-right: [w46] -> _
    shift-left: _ -> [w48]
    tunnel: w2 -> [w43]
    tunnel: w3 -> [w38]
    stop <- w39 stop-if-true
    n19 = Preview Queue Element(queue=w43) -> (queue out=w40:refnum<queue>, element=w45:string)  [unwired: 2 in, 2 out]
    n20 = Match Pattern(string=w45, regular expression=":") -> (before substring=w42:string, after substring=w41:string)  [unwired: 1 in, 2 out]
    n21 = case shown="\"single\"" w42 {
      tunnel: w52 -> [_ _ w85 _ w256 w359]
      tunnel: w51 -> [_ _ w84 _ _ _]
      tunnel: w50 -> [_ _ w83 _ w255 w361]
      tunnel: w49 -> [w54 w58 _ w216 w252 w358]
      tunnel: w48 -> [w53 w57 _ w215 w251 w357]
      tunnel: [w54 w58 w82 w216 w252 w358] -> w47
      tunnel: [w53 w57 w65 w215 w251 w357] -> w46
      tunnel: w41 -> [_ _ _ _ _ _]
      tunnel: w40 -> [w56 _ w74 w219 w250 w360]
      tunnel: [TRUE _ _ _ _ _] -> w39
      tunnel: w38 -> [_ _ _ _ w254 _]
      frame "close" {
        n22 = Release Queue(queue=w56) -> ()  [unwired: 2 in, 3 out]
      }
      frame "idle", Default {
      }
      frame "GO" {
        n23 = Dequeue Element(queue=w74) -> (queue out=w73:refnum<queue>)  [unwired: 2 in, 3 out]
        n24 = local read "RunNumber"() -> (w80:u16)
        n25 = local read "BasePath"() -> (w79:path)
        n26 = local read "ESP Axis"() -> (w77:i32)
        n27 = local read "ESP_t0"() -> (w63:dbl)
        n28 = Increment(x=w80) -> (x+1=w78:u16)
        n29 = Current VI's Path() -> (path=w81:path)
        n30 = call "2delaypoints.vi"("Offset (mm)"=w63, "delay table [fs]"="delay table [fs]") -> ("delay points [mm]"=w62:dbl[], "delay pointss [fs]"=w60:dbl[])
        n31 = Number To Decimal String(number=w77) -> (decimal integer string=w76:string)  [unwired: 1 in]
        n32 = call "create_opti_path.vi"("RunNumber"=w78, "base path"=w79) -> ("Path"=w70:path)  [unwired: 2 in]
        n33 = call "saverunnumber.vi"("RunNumber"=w78, "VI path"=w81) -> ()  [unwired: 10 in]
        n34 = local write "RunNumber"(w78) -> ()
        n35 = Get Date/Time In Seconds() -> (seconds since 1Jan1904=w59:timestamp)
        n36 = Build Path(base path=w70, name or relative path="info.txt") -> (appended path=w61:path)
        n37 = while {
          tunnel: w62 -> [w122]
          tunnel: w76 -> [w130]
          tunnel: w84 -> [w129]
          tunnel: w85 -> [w128]
          tunnel: w73 -> [w127]
          tunnel: w83 -> [w126]
          tunnel: w70 -> [w125]
          shift-right: [w123] -> w82
          shift-left: dbl[][][] [] -> [w124]
          tunnel: [w121] -> w66
          tunnel: w61 -> [w88]
          tunnel: w60 -> [w87]
          tunnel: w59 -> [w86]
          i -> [w120]
          stop <- w116 stop-if-true
          n38 = for {
            N -> [w149]
            tunnel: w122 -> [w158] mode=indexing
            tunnel: w130 -> [w175]
            tunnel: w129 -> [w174]
            tunnel: w128 -> [w169]
            tunnel: w127 -> [w173]
            tunnel: w126 -> [w172]
            tunnel: w125 -> [w143]
            shift-right: [w133] -> w123
            shift-left: w124 -> [w165]
            tunnel: w120 -> [w142]
            tunnel: w87 -> [w132]
            tunnel: [w132] -> w121
            tunnel: [w155] -> w118
            tunnel: w86 -> [w145]
            tunnel: "delscan_iters" -> [w150]
            i -> [w135]
            stop <- "delscan_abort" stop-if-true
            w177 = ":" ("string")
            # "average data"
            # "init array?"
            n39 = Number To Fractional String(number=w158) -> (F-format string=w167:string)  [unwired: 3 in]
            n40 = property on="delscan_progress" class="Slide (strict)"("Scale.Maximum"=w149) -> ()  [unwired: 2 in, 2 out]
            n41 = Get Date/Time In Seconds() -> (seconds since 1Jan1904=w153:timestamp)
            n42 = call "createFileStruc.vi"("i_iter"=w142, "i_delay"=w135, "meas_path"=w143) -> ("AVG file"=w138:path, "RAW file"=w139:path)  [unwired: 7 in]
            n43 = Concatenate Strings("abs:" ("string"), w175, w177, w167, w177, "wait" ("string")) -> (w180:string)
            n44 = Enqueue Element(queue=w174, element=w180) -> (error out=w178:errorcluster)  [unwired: 2 in, 2 out]
            n45 = Subtract(x=w153, y=w145) -> (x-y=w151:dbl)
            n46 = Equal To 0?(x=w135) -> (x = 0?=w141:bool)
            n47 = Equal To 0?(x=w142) -> (x = 0?=w140:bool)
            n48 = Dequeue Element(queue=w173, error in (no error)=w178) -> (error out=w170:errorcluster)  [unwired: 1 in, 3 out]
            n49 = And(x=w141, y=w140) -> (x .and. y?=w166:bool)
            n50 = Enqueue Element(queue=w172, element="snap", error in (no error)=w170) -> (error out=w168:errorcluster)  [unwired: 1 in, 2 out]
            n51 = Dequeue Element(queue=w169, error in (no error)=w168) -> (element=w161:dbl[][])  [unwired: 1 in, 3 out]
            n52 = Multiply(x=w149, y=w142) -> (x*y=w154:i32)
            n53 = Multiply(x=w149, y=w150) -> (x*y=w148:u32)
            n54 = Array Size(array=w161) -> (size(s)=w162:i32[])
            n55 = Add(x=w154, y=w135) -> (x+y=w152:i32)
            n56 = call-poly <vilib>:"Write Delimited Spreadsheet.vi"("file path (dialog if empty)"=w139, "2D data"=w161) -> ()  [unwired: 12 in, 2 out]
            n57 = Index Array(array=w162) -> (element #1=w160:i32, element #2=w159:i32)  [unwired: 2 in]
            n58 = Divide(x=w151, y=w152) -> (x/y=w147:dbl)
            "time / step" <- w147
            n59 = Multiply(x=w148, y=w147) -> (x*y=w146:dbl)
            n60 = case shown="True" w166 {
              tunnel: w149 -> [_ w188]
              tunnel: [w183 w186] -> w164
              tunnel: w165 -> [w183 _]
              tunnel: w160 -> [_ w185]
              tunnel: w159 -> [_ w184]
              frame False {
              }
              frame True {
                n61 = Initialize Array(0.0 ("element"), w188, w185, w184) -> (w186:dbl[][][])
              }
            }
            n62 = Add(x=w145, y=w146) -> (x+y=→"del_ETA":timestamp)
            n63 = for {
              N: w160 -> [_]
              tunnel: w135 -> [w195]
              shift-right: [w193] -> w133
              shift-left: w164 -> [w196]
              tunnel: w142 -> [w191]
              shift-right: [w190] -> w163
              shift-left: w161 -> [w192]
              tunnel: w159 -> [w189]
              i -> [w194]
              n64 = for {
                N: w189 -> [_]
                tunnel: w195 -> [w203]
                tunnel: w194 -> [w200]
                shift-right: [w202] -> w193
                shift-left: w196 -> [w204]
                tunnel: w191 -> [w198]
                shift-right: [w197] -> w190
                shift-left: w192 -> [w201]
                i -> [w199]
                n65 = in-place {
                  in-place-border: w198 -> [w210]
                  n66 = in-place-array #1(w204, w203, w200, w199) -> (w211:dbl)
                  n67 = in-place-array #2(w201, w200, w199) -> (w208:dbl)
                  n68 = Multiply(x=w211, y=w210) -> (x*y=w209:dbl)
                  n69 = Increment(x=w210) -> (x+1=w206:i32)
                  n70 = Add(x=w209, y=w208) -> (x+y=w207:dbl)
                  n71 = Divide(x=w207, y=w206) -> (x/y=w205:dbl)
                  n72 = in-place-array #1(w205) -> (w202:dbl[][][])  [unwired: 3 out]
                  n73 = in-place-array #2(w205) -> (w197:dbl[][])  [unwired: 2 out]
                }
              }
            }
            n74 = call-poly <vilib>:"Write Delimited Spreadsheet.vi"("file path (dialog if empty)"=w138, "2D data"=w163) -> ()  [unwired: 12 in, 2 out]
            n75 = property on="mainimg" class="IntGraph (strict)"() -> ("CrsrLis"=w134:T4)  [unwired: 2 in, 2 out]
            n76 = Increment(x=w135) -> (x+1=w136:i32)
            n77 = call "processData.vi"("Cursor List"=w134, "data in"=w133, "scan vector"=w132) -> ("output cluster"=w131:cluster{"scan vector":dbl[], dbl[]})
            n78 = flat-sequence {
              tunnel: w131 -> [w182]
              tunnel: [w182] -> w137
              tunnel: w136 -> [w181]
              frame #0 {
                "delscan_progress" <- w181
              }
            }
            n79 = Or(x="delscan_finishIteration", y="delscan_abort") -> (x .or. y?=w155:bool)
            "delscan_pos" <- w158
            "scangraph" <- w137
          }
          n80 = Increment(x=w120) -> (x+1=w119:i32)
          "iteration" <- w119
          n81 = local read "exposure [ms]"() -> (w103:u32)
          n82 = local read "delscan_iters"() -> (w113:u32)
          n83 = local read "ROI Bottom"() -> (w106:i32)
          n84 = property on="Mode" class="Enum (strict)"() -> ("RingText.Text"=w92:string)  [unwired: 2 in, 2 out]
          n85 = property on="VoltageRange" class="Enum (strict)"() -> ("RingText.Text"=w93:string)  [unwired: 2 in, 2 out]
          n86 = local read "cam_dark?"() -> (w90:bool)
          n87 = local read "phoib_I_1"() -> (w94:dbl)
          n88 = local read "phoib_I_2"() -> (w95:dbl)
          n89 = local read "phoib_I_3"() -> (w96:dbl)
          n90 = local read "phoib_I_4"() -> (w97:dbl)
          n91 = local read "phoib_I_5"() -> (w98:dbl)
          n92 = local read "phoib_I_6"() -> (w99:dbl)
          n93 = local read "phoib_I_7"() -> (w100:dbl)
          n94 = local read "phoib_I_8"() -> (w101:dbl)
          n95 = local read "phoib_I_9"() -> (w102:dbl)
          n96 = local read "ROI Right"() -> (w108:i32)
          n97 = local read "averages"() -> (w112:i32)
          n98 = local read "ROI Top"() -> (w107:i32)
          n99 = local read "ROI Left"() -> (w109:i32)
          n100 = local read "binning"() -> (w105:u16)
          n101 = local read "ESP_t0"() -> (w114:dbl)
          n102 = local read "gain"() -> (w89:bool)
          n103 = Boolean To (0,1)(Boolean=w89) -> (0, 1=w104:i16)
          n104 = Boolean To (0,1)(Boolean=w90) -> (0, 1=w110:i16)
          n105 = Format Into String(format string="ScanType:%s\\nAverages:%u\\nRepetitions:%u\\nTimeZero:%f\\nLensMode:%s\\nVoltageRange:%s\\nKineticEnergy:%f\\nPassEnergy:%f\\nCoilCurrent:%f\\nWorkFunction:%f\\nDetectorVoltage:%f\\nScreenVoltage:%f\\nConversionVoltage:%f\\nFocusDisplacement1:%f\\nFocusDisplacement2:%f\\nExposure:%u\\nGain:%u\\nBinning:%u\\nROIbottom:%u\\nROItop:%u\\nROIright:%u\\nROIleft:%u\\nDarkImg:%u\\nStartTime:%<%Y.%m.%d %H:%M:%S>T", initial string=w88, "delay" ("input 1"), w112, w113, w114, w92, w93, w94, w95, w96, w97, w98, w99, w100, w101, w102, w103, w104, w105, w106, w107, w108, w109, w110, w86) -> ()  [unwired: 1 in, 2 out]
          n106 = Less Or Equal?(x="delscan_iters", y=w119) -> (x <= y?=w117:bool)
          n107 = Or(x=w118, y=w117) -> (x .or. y?=w116:bool)
        }
        n108 = Build Path(base path=w70, name or relative path="scanvector.txt") -> (appended path=w67:path)
        n109 = call-poly <vilib>:"Write Delimited Spreadsheet.vi"("file path (dialog if empty)"=w67, "format (%.3f)"="%.6f", "1D data"=w62, "transpose? (no:F)"=TRUE ("transpose? (F)")) -> ()  [unwired: 10 in, 2 out]
        n110 = flat-sequence {
          tunnel: w66 -> [w214]
          tunnel: [w214] -> w65
          frame #0 {
            w213 = u32 1000 ("frequency (Hz)")
            n111 = call <vilib>:"Beep.vi"("use system alert? (T)"=FALSE, "duration (msec)"=w213, "frequency (Hz)"=w213) -> ()  [unwired: 9 in]
          }
        }
      }
      frame "refresh" {
        n112 = Dequeue Element(queue=w219) -> ()  [unwired: 2 in, 4 out]
        n113 = property on="mainimg" class="IntGraph (strict)"() -> ("CrsrLis"=w218:T4)  [unwired: 2 in, 2 out]
        n114 = call "processData.vi"("Cursor List"=w218, "data in"=w216, "scan vector"=w215) -> ("output cluster"=w217:cluster{"scan vector":dbl[], dbl[]})
        n115 = local write "scangraph"(w217) -> ()
      }
      frame "manip" {
        n116 = Dequeue Element(queue=w250) -> (queue out=w249:refnum<queue>)  [unwired: 2 in, 3 out]
        n117 = local read "RunNumber"() -> (w258:u16)
        n118 = local read "BasePath"() -> (w259:path)
        n119 = property on="delscan_progress 2" class="Slide (strict)"("Scale.Maximum"="manip_scan_steps") -> ()  [unwired: 2 in, 2 out]
        n120 = Index Array(array="manip_scan_delta") -> (element #1=w271:dbl, element #2=w270:dbl, element #3=w269:dbl, element #4=w268:dbl, element #5=w267:dbl, element #6=w266:dbl)  [unwired: 6 in]
        n121 = Increment(x=w258) -> (x+1=w260:u16)
        n122 = Current VI's Path() -> (path=w257:path)
        n123 = Format Into String(format string="%g_%g_%g_%g_%g_%g", w271, w270, w269, w268, w267, w266) -> (resulting string=w264:string)  [unwired: 2 in, 1 out]
        n124 = property on="Mode" class="Enum (strict)"() -> ("RingText.Text"=w244:string)  [unwired: 2 in, 2 out]
        n125 = property on="VoltageRange" class="Enum (strict)"() -> ("RingText.Text"=w243:string)  [unwired: 2 in, 2 out]
        n126 = call "saverunnumber.vi"("RunNumber"=w260, "VI path"=w257) -> ()  [unwired: 10 in]
        n127 = local write "RunNumber"(w260) -> ()
        n128 = call "create_opti_path.vi"("RunNumber"=w260, "base path"=w259) -> ("Path"=w223:path)  [unwired: 2 in]
        n129 = local read "exposure [ms]"() -> (w233:u32)
        n130 = Build Path(base path=w223, name or relative path="info.txt") -> (appended path=w222:path)
        n131 = Concatenate Strings("relative:" ("string"), w264, ":wait" ("string")) -> (w273:string)
        n132 = local read "ROI Bottom"() -> (w230:i32)
        n133 = local read "cam_dark?"() -> (w247:bool)
        n134 = local read "phoib_I_1"() -> (w242:dbl)
        n135 = local read "phoib_I_2"() -> (w241:dbl)
        n136 = local read "phoib_I_3"() -> (w240:dbl)
        n137 = local read "phoib_I_4"() -> (w239:dbl)
        n138 = local read "phoib_I_5"() -> (w238:dbl)
        n139 = local read "phoib_I_6"() -> (w237:dbl)
        n140 = local read "phoib_I_7"() -> (w236:dbl)
        n141 = local read "phoib_I_8"() -> (w235:dbl)
        n142 = local read "phoib_I_9"() -> (w234:dbl)
        n143 = local read "ROI Right"() -> (w228:i32)
        n144 = local read "averages"() -> (w245:i32)
        n145 = local read "ROI Top"() -> (w229:i32)
        n146 = local read "ROI Left"() -> (w227:i32)
        n147 = local read "binning"() -> (w231:u16)
        n148 = local read "gain"() -> (w248:bool)
        n149 = Get Date/Time In Seconds() -> (seconds since 1Jan1904=w225:timestamp)
        n150 = Build Path(base path=w223, name or relative path="scanvector.txt") -> (appended path=w274:path)
        n151 = for {
          N: 1 -> [_]
          tunnel: w256 -> [w289]
          tunnel: w223 -> [w288]
          tunnel: w274 -> [w281]
          tunnel: "manip_scan_steps" -> [w280]
          tunnel: w273 -> [w279]
          tunnel: w254 -> [w278]
          tunnel: w249 -> [w277]
          tunnel: w255 -> [w276]
          tunnel: "manip_scan_delta" -> [w275]
          i -> [w283]
          n152 = Add(x=w283, y=1000) -> (x+y=w286:i32)
          n153 = Number To Decimal String(number=w286) -> (decimal integer string=w285:string)  [unwired: 1 in]
          n154 = String Subset(string=w285, offset (0)=1) -> (substring=w282:string)  [unwired: 1 in]
          n155 = for {
            N: w280 -> [_]
            tunnel: w289 -> [w312]
            tunnel: w288 -> [w309]
            tunnel: w282 -> [w303]
            tunnel: w281 -> [w305]
            tunnel: w279 -> [w300]
            tunnel: w278 -> [w299]
            tunnel: w277 -> [w298]
            tunnel: w276 -> [w297]
            tunnel: w275 -> [w295]
            i -> [w290]
            stop <- "abort" stop-if-true
            n156 = Increment(x=w290) -> (x+1=→"delscan_progress 2":i32)
            n157 = Multiply(x=w295, y=w290) -> (x*y=w294:dbl[])
            n158 = Enqueue Element(queue=w299, element=w300) -> (error out=w301:errorcluster)  [unwired: 2 in, 2 out]
            n159 = Add(x=w290, y=10000) -> (x+y=w318:i32)
            n160 = Dequeue Element(queue=w298, error in (no error)=w301) -> (error out=w296:errorcluster)  [unwired: 1 in, 3 out]
            n161 = Number To Decimal String(number=w318) -> (decimal integer string=w317:string)  [unwired: 1 in]
            n162 = String Subset(string=w317, offset (0)=1) -> (substring=w302:string)  [unwired: 1 in]
            n163 = Enqueue Element(queue=w297, element="snap", error in (no error)=w296) -> (error out=w311:errorcluster)  [unwired: 1 in, 2 out]
            n164 = Concatenate Strings("RAW\\" ("string"), w303, "_" ("string"), w302, ".tsv" ("string")) -> (w308:string)
            n165 = Dequeue Element(queue=w312, error in (no error)=w311) -> (element=w307:dbl[][])  [unwired: 1 in, 3 out]
            n166 = Build Path(base path=w309, name or relative path=w308) -> (appended path=w310:path)
            n167 = call-poly <vilib>:"Write Delimited Spreadsheet.vi"("file path (dialog if empty)"=w310, "2D data"=w307) -> ()  [unwired: 12 in, 2 out]
            n168 = call-poly <vilib>:"Write Delimited Spreadsheet.vi"("file path (dialog if empty)"=w305, "1D data"=w294, "append to file? (new file:F)"=TRUE ("append to file? (F)"), "transpose? (no:F)"=FALSE ("transpose? (F)")) -> ()  [unwired: 10 in, 2 out]
          }
        }
        n169 = Boolean To (0,1)(Boolean=w248) -> (0, 1=w232:i16)
        n170 = Boolean To (0,1)(Boolean=w247) -> (0, 1=w226:i16)
        n171 = Format Into String(format string="ScanType:%s\\nAverages:%u\\nMode:%s\\nVoltageRange:%s\\nKineticEnergy:%f\\nPassEnergy:%f\\nCoilCurrent:%f\\nWorkFunction:%f\\nDetectorVoltage:%f\\nScreenVoltage:%f\\nConversionVoltage:%f\\nFocusDisplacement1:%f\\nFocusDisplacement2:%f\\nExposure:%u\\nGain:%u\\nBinning:%u\\nROIbottom:%u\\nROItop:%u\\nROIright:%u\\nROIleft:%u\\nDarkImg:%u\\nStartTime:%<%Y.%m.%d %H:%M:%S>T", initial string=w222, "manipulator" ("input 1"), w245, w244, w243, w242, w241, w240, w239, w238, w237, w236, w235, w234, w233, w232, w231, w230, w229, w228, w227, w226, w225) -> ()  [unwired: 1 in, 2 out]
      }
      frame "single" {
        n172 = Dequeue Element(queue=w360) -> ()  [unwired: 2 in, 4 out]
        n173 = property on="Mode" class="Enum (strict)"() -> ("RingText.Text"=w347:string)  [unwired: 2 in, 2 out]
        n174 = property on="VoltageRange" class="Enum (strict)"() -> ("RingText.Text"=w346:string)  [unwired: 2 in, 2 out]
        n175 = local read "RunNumber"() -> (w351:u16)
        n176 = local read "BasePath"() -> (w352:path)
        n177 = local read "exposure [ms]"() -> (w336:u32)
        n178 = local read "ROI Bottom"() -> (w333:i32)
        n179 = local read "cam_dark?"() -> (w348:bool)
        n180 = local read "phoib_I_1"() -> (w345:dbl)
        n181 = local read "phoib_I_2"() -> (w344:dbl)
        n182 = local read "phoib_I_3"() -> (w343:dbl)
        n183 = local read "phoib_I_4"() -> (w342:dbl)
        n184 = local read "phoib_I_5"() -> (w341:dbl)
        n185 = local read "phoib_I_6"() -> (w340:dbl)
        n186 = local read "phoib_I_7"() -> (w339:dbl)
        n187 = local read "phoib_I_8"() -> (w338:dbl)
        n188 = local read "phoib_I_9"() -> (w337:dbl)
        n189 = local read "ROI Right"() -> (w331:i32)
        n190 = local read "averages"() -> (w321:i32)
        n191 = local read "ROI Top"() -> (w332:i32)
        n192 = local read "ROI Left"() -> (w330:i32)
        n193 = local read "binning"() -> (w334:u16)
        n194 = Increment(x=w351) -> (x+1=w353:u16)
        n195 = Current VI's Path() -> (path=w350:path)
        n196 = local read "gain"() -> (w349:bool)
        n197 = Get Date/Time In Seconds() -> (seconds since 1Jan1904=w328:timestamp)
        n198 = call "saverunnumber.vi"("RunNumber"=w353, "VI path"=w350) -> ()  [unwired: 10 in]
        n199 = local write "RunNumber"(w353) -> ()
        n200 = call "create_opti_path.vi"("RunNumber"=w353, "base path"=w352) -> ("Path"=w325:path)  [unwired: 2 in]
        n201 = Boolean To (0,1)(Boolean=w349) -> (0, 1=w335:i16)
        n202 = Boolean To (0,1)(Boolean=w348) -> (0, 1=w329:i16)
        n203 = Build Path(base path=w325, name or relative path="info.txt") -> (appended path=w323:path)
        n204 = Format Into String(format string="ScanType:%s\\nAverages:%u\\nMode:%s\\nVoltageRange:%s\\nKineticEnergy:%f\\nPassEnergy:%f\\nCoilCurrent:%f\\nWorkFunction:%f\\nDetectorVoltage:%f\\nScreenVoltage:%f\\nConversionVoltage:%f\\nFocusDisplacement1:%f\\nFocusDisplacement2:%f\\nExposure:%u\\nGain:%u\\nBinning:%u\\nROIbottom:%u\\nROItop:%u\\nROIright:%u\\nROIleft:%u\\nDarkImg:%u\\nStartTime:%<%Y.%m.%d %H:%M:%S>T", initial string=w323, "single" ("input 1"), w321, w347, w346, w345, w344, w343, w342, w341, w340, w339, w338, w337, w336, w335, w334, w333, w332, w331, w330, w329, w328) -> ()  [unwired: 1 in, 2 out]
        n205 = Build Path(base path=w325, name or relative path="AVG\\000.tsv") -> (appended path=w326:path)
        n206 = Enqueue Element(queue=w361, element="snap" ("string")) -> (error out=w355:errorcluster)  [unwired: 2 in, 2 out]
        n207 = Dequeue Element(queue=w359, error in (no error)=w355) -> (element=w354:dbl[][])  [unwired: 1 in, 3 out]
        n208 = call-poly <vilib>:"Write Delimited Spreadsheet.vi"("file path (dialog if empty)"=w326, "2D data"=w354) -> ()  [unwired: 12 in, 2 out]
      }
    }
  }
  n209 = while {
    tunnel: w10 -> [w386]
    shift-right: [w380] -> _
    shift-left: _ -> [w379]
    shift-right: [w378] -> _
    shift-left: _ -> [w376]
    shift-right: [w377] -> _
    shift-left: _ -> [w375]
    shift-right: [w372] -> _
    shift-left: 0 -> [w373]
    shift-right: [w371] -> _
    shift-left: _ -> [w370]
    shift-right: [w369] -> _
    shift-left: _ -> [w368]
    tunnel: w11 -> [w367]
    shift-right: [w366] -> _
    shift-left: _ -> [w365]
    shift-right: [w363] -> _
    shift-left: _ -> [w362]
    i -> [w364]
    stop <- w374 stop-if-true
    # "cam"
    n210 = Preview Queue Element(queue=w386, timeout in ms (-1)=w373) -> (queue out=w385:refnum<queue>, element=w384:string)  [unwired: 1 in, 2 out]
    n211 = Match Pattern(string=w384, regular expression=":") -> (before substring=w381:string, after substring=w382:string)  [unwired: 1 in, 2 out]
    n212 = case shown="\"snap\"" w381 {
      tunnel: w385 -> [w396 w426 w454 w466 _ w552 w580 w643]
      tunnel: w382 -> [_ _ _ _ _ _ _ _]
      tunnel: [w390 w412 w453 w464 w506 w549 w569 w641] -> w380
      tunnel: w379 -> [_ _ w453 w464 w506 w549 w569 w641]
      tunnel: [w395 w427 u64 0 ("Hout") w463 w510 w550 w575 w640] -> w378
      tunnel: [w397 w428 w450 w462 w511 w551 w563 w639] -> w377
      tunnel: w376 -> [_ w430 w452 w463 w513 w554 w577 w640]
      tunnel: w375 -> [_ w429 _ w462 w512 w553 w576 w639]
      tunnel: [_ _ _ TRUE _ _ _ _] -> w374
      tunnel: [_ _ _ _ _ _ _ -1] -> w372
      tunnel: [w389 w413 _ _ w520 _ _ _] -> w371
      tunnel: w370 -> [w389 w413 _ _ w519 _ _ _]
      tunnel: [w390 w415 w448 w461 w515 w543 w578 w638] -> w369
      tunnel: w368 -> [_ w415 w448 w461 w515 _ w578 w638]
      tunnel: w367 -> [_ _ _ _ _ _ w567 _]
      tunnel: [w387 w410 w447 w459 w473 w540 w572 w637] -> w366
      tunnel: w365 -> [w387 w410 w447 w459 w508 w540 w572 w637]
      tunnel: w364 -> [_ _ _ _ w481 _ _ _]
      tunnel: [w388 w411 w446 w460 w507 w539 w571 w636] -> w363
      tunnel: w362 -> [w388 w411 w446 w460 w480 w539 w571 w636]
      frame "init" {
        w390 = u16[][] []
        n213 = flat-sequence {
          tunnel: [w399] -> w394
          tunnel: [w400] -> w393
          tunnel: [w408] -> w395
          tunnel: [w409] -> w397
          tunnel: w394 -> [w409]
          tunnel: w393 -> [w408]
          frame #0 {
            n214 = local write "cam_con?"(FALSE ("cam_con?")) -> ()
          }
          frame #1 {
            n215 = call "SCInitBoard.vi"("boardnr"="board number") -> ("Hout"=w403:u32, "error out"=w404:errorcluster)  [unwired: 1 in, 1 out]
            n216 = call "SCSetupCamera.vi"("Handle"=w403, "error in (no error)"=w404) -> ("Hout"=w405:u64, "error out"=w406:errorcluster)  [unwired: 1 out]
            n217 = call "SCStopCOC.vi"("error in (no error)"=w406, "Stop mode"=0, "Handle"=w405) -> ("error out"=w399:errorcluster, "Hout"=w400:u64)
          }
          frame #2 {
            n218 = local write "cam_con?"(TRUE ("cam_con?")) -> ()
          }
        }
        n219 = Dequeue Element(queue=w396) -> (queue out=w392:refnum<queue>)  [unwired: 2 in, 3 out]
        n220 = Enqueue Element At Opposite End(queue=w392, element="set") -> ()  [unwired: 2 in, 3 out]
      }
      frame "set" {
        w425 = u32 1 ("Operating mode\nHP & QE / HS & DiCam Pro")
        n221 = Dequeue Element(queue=w426) -> ()  [unwired: 2 in, 4 out]
        n222 = Bundle By Name(cluster=cluster{"Delay":dbl, "Exposure ":dbl} {"Delay"=0.0, "Exposure "=0.0} ("Delay and exposure"), "Exposure"="exposure [ms]") -> (w422:cluster{"Delay":dbl, "Exposure ":dbl})
        n223 = call "SCStopCOC.vi"("error in (no error)"=w429, "Stop mode"=0, "Handle"=w430) -> ("error out"=w445:errorcluster, "Hout"=w444:u64)
        n224 = Bundle By Name(cluster=T5 {"Camera type"=0, "Operating mode\nHP & QE / HS & DiCam Pro "=0, "Frame trigger \n(High Performance and QE only)"=0, "Sequence trigger"=0, "Low Light\n(QE only)"=FALSE, "Gain"=FALSE, "Horzontal\nbinning"=0, "Vertical\nbinning "=0, "ROI Left"=1, "ROI Right"=20, "ROI Top"=1, "ROI Bottom"=15} ("Camera controls"), "Operating mode\nHP & QE / HS & DiCam Pro"=w425, "Horzontal\nbinning"="binning", "Vertical\nbinning"="binning", "ROI Left"="ROI Left", "ROI Right"="ROI Right", "ROI Top"="ROI Top", "ROI Bottom"="ROI Bottom", "Gain"="gain") -> (w440:T5)
        n225 = call "New delay and exposure forma.vi"("Operating mode\nHP & QE / HS & DiCam Pro"=w425, "Delay and exposure"=w422) -> ("Output table"=w441:string)  [unwired: 3 in]
        n226 = call "SCSetCoC.vi"("error in (no error)"=w445, "Delay and exposure table"=w441, "Camera controls"=w440, "Handle"=w444) -> ("error out"=w433:errorcluster, "Hout"=w432:u64)  [unwired: 1 out]
        n227 = call "SCGetImageSize.vi"("Handle"=w432, "error in (no error)"=w433) -> ("Hout"=w431:u64, "error out"=w414:errorcluster, "Horizontal size"=w419:i32, "Vertical size"=w418:i32)  [unwired: 2 out]
        n228 = Greater?(x=w419, y=w418) -> (0:w420:bool)
        n229 = Initialize Array(u16 0 ("dimension size"), w418, w419) -> (w412:u16[][])
        n230 = call "SCRun.vi"("error in (no error)"=w414, "Run mode"=0, "Handle"=w431) -> ("error out"=w428:errorcluster, "Hout"=w427:u64)  [unwired: 1 out]
        n231 = Select(t=w419, s=w420, f=w418) -> (s? t:f=w417:i32)
        n232 = property on="mainimg" class="IntGraph (strict)"("XScale.Maximum"=w417, "YScale.Maximum"=w417) -> ()  [unwired: 2 in, 2 out]
      }
      frame "release" {
        n233 = Dequeue Element(queue=w454) -> ()  [unwired: 2 in, 4 out]
        n234 = flat-sequence {
          tunnel: w452 -> [w456]
          tunnel: [w455] -> w449
          tunnel: [w458] -> w450
          tunnel: w449 -> [w458]
          frame #0 {
            n235 = call "SCCloseBoard.vi"("Handle"=w456) -> ("error out"=w455:errorcluster)  [unwired: 1 in, 2 out]
          }
          frame #1 {
            n236 = local write "cam_con?"(FALSE ("cam_con?")) -> ()
          }
        }
      }
      frame "close" {
        n237 = Release Queue(queue=w466) -> ()  [unwired: 2 in, 3 out]
      }
      frame "idle", Default {
        n238 = call "grabimg.vi"("array in"=w506, "error in"=w512, "Hin"=w513) -> ("error out"=w511:errorcluster, "imgdata"=w509:i32[][], "Hout"=w510:u64)  [unwired: 6 in]
        n239 = local read "lower threshold"() -> (w504:i32)
        n240 = case shown="False" "cam_dark?" {
          tunnel: w515 -> [_ w538]
          tunnel: [w535 w537] -> w505
          tunnel: w509 -> [w535 w536]
          frame False {
          }
          frame True {
            n241 = Subtract(x=w536, y=w538) -> (x-y=w537:dbl[][])
          }
        }
        n242 = call "filtr_b.vi"("threshold"=w504, "input array"=w505) -> ("output array"=w496:dbl[][])  [unwired: 9 in]
        n243 = call <vilib>:"High Resolution Relative Seconds.vi"() -> ("relative seconds"=w520:dbl)
        n244 = Subtract(x=w520, y=w519) -> (x-y=w518:dbl)
        n245 = Array Size(array=w496) -> (size(s)=w495:i32[])
        n246 = Reciprocal(x=w518) -> (1/x=→"cam_fps":dbl)
        n247 = Index Array(array=w495) -> (element #1=w490:i32, element #2=w489:i32)  [unwired: 2 in]
        n248 = Subtract(x=w481, y=w480) -> (x-y=w479:i32)
        n249 = Less Or Equal?(x="pics2avg", y=w479) -> (x <= y?=w502:bool)
        n250 = And(x="reset every n pics", y=w502) -> (x .and. y?=w500:bool)
        n251 = Not(x=w500) -> (.not. x?=w499:bool)
        n252 = call-poly <vilib>:"Ramp Pattern.vi"("start"=0.0, "end"=w490, "samples"=w490) -> ("Ramp Pattern"=w485:dbl[])  [unwired: 7 in, 1 out]
        n253 = call-poly <vilib>:"Ramp Pattern.vi"("start"=0.0, "end"=w489, "samples"=w489) -> ("Ramp Pattern"=w486:dbl[])  [unwired: 7 in, 1 out]
        n254 = property on="mainimg" class="IntGraph (strict)"() -> ("CrsrLis"=w478:T4)  [unwired: 2 in, 2 out]
        n255 = And(x="cam_liveavg", y=w499) -> (x .and. y?=w497:bool)
        n256 = case shown="False" w497 {
          tunnel: w496 -> [w525 w531]
          tunnel: [w525 w528] -> w473
          tunnel: w508 -> [_ w533]
          tunnel: w481 -> [w526 _]
          tunnel: [w526 w534] -> w507
          tunnel: w480 -> [_ w534]
          tunnel: w479 -> [_ w527]
          frame False {
          }
          frame True {
            n257 = Multiply(x=w533, y=w527) -> (x*y=w532:dbl[][])
            n258 = Increment(x=w527) -> (x+1=w529:i32)
            n259 = Add(x=w532, y=w531) -> (x+y=w530:dbl[][])
            n260 = Divide(x=w530, y=w529) -> (x/y=w528:dbl[][])
          }
        }
        "mainimg" <- w473
        n261 = Index Array(array=w478) -> (element #1=w476:T6, element #2=w477:T6)  [unwired: 2 in]
        n262 = Unbundle By Name(w476) -> ("Position.X"=w470:dbl, "Position.Y"=w472:dbl)
        n263 = Unbundle By Name(w477) -> ("Position.X"=w474:dbl, "Position.Y"=w475:dbl)
        n264 = Array Max & Min(array=w473) -> (max value=→"max":dbl)  [unwired: 3 out]
        n265 = Subtract(x=w475, y=w472) -> (x-y=w471:dbl)
        n266 = Subtract(x=w474, y=w470) -> (x-y=w469:dbl)
        n267 = Array Subset(array=w473, index (row)=w472, length (row)=w471) -> (w484:dbl[][])  [unwired: 2 in]
        n268 = Array Subset(array=w473, index (col)=w470, length (col)=w469) -> (w482:dbl[][])  [unwired: 2 in]
        n269 = Array Subset(array=w473, index (row)=w472, length (row)=w471, index (col)=w470, length (col)=w469) -> (w468:dbl[][])
        n270 = Transpose 2D Array(2D array=w484) -> (transposed array=w483:dbl[][])
        n271 = Add Array Elements(numeric array=w468) -> (sum=→"sum" →"Waveform Chart":dbl)
        n272 = for {
          tunnel: w482 -> [w522] mode=indexing
          tunnel: [w521] -> w492 mode=indexing
          n273 = Add Array Elements(numeric array=w522) -> (sum=w521:dbl)
        }
        n274 = for {
          tunnel: w483 -> [w524] mode=indexing
          tunnel: [w523] -> w491 mode=indexing
          n275 = Add Array Elements(numeric array=w524) -> (sum=w523:dbl)
        }
        n276 = Bundle("Ramp Pattern"=w486, w491) -> (→"G2 X":cluster{"Ramp Pattern":dbl[], dbl[]})  [unwired: 1 in]
        n277 = Bundle(w492, "Ramp Pattern"=w485) -> (→"G2 Y":cluster{dbl[], "Ramp Pattern":dbl[]})  [unwired: 1 in]
      }
      frame "dark" {
        n278 = Dequeue Element(queue=w552) -> ()  [unwired: 2 in, 4 out]
        n279 = Array Size(array=w549) -> (size(s)=w548:i32[])
        n280 = Index Array(array=w548) -> (element #1=w547:i32, element #2=w546:i32)  [unwired: 2 in]
        n281 = Initialize Array(0.0 ("element"), w547, w546) -> (w544:dbl[][])
        n282 = for {
          N: "dark avg" -> [_]
          tunnel: w554 -> [w562]
          tunnel: w553 -> [w561]
          tunnel: [w560] -> w551
          tunnel: w549 -> [w559]
          tunnel: [w558] -> w550
          shift-right: [w555] -> w542
          shift-left: w544 -> [w556]
          n283 = call "grabimg.vi"("array in"=w559, "error in"=w561, "Hin"=w562) -> ("error out"=w560:errorcluster, "imgdata"=w557:i32[][], "Hout"=w558:u64)  [unwired: 6 in]
          n284 = Add(x=w557, y=w556) -> (x+y=w555:dbl[][])
        }
        n285 = Divide(x=w542, y="dark avg") -> (x/y=w543:dbl[][])
      }
      frame "snap" {
        n286 = Dequeue Element(queue=w580) -> ()  [unwired: 2 in, 4 out]
        n287 = local read "cam_dark?"() -> (w579:bool)
        n288 = local read "averages"() -> (w574:i32)
        n289 = To Double Precision Float(number=w569) -> (double precision float=w568:dbl[][])
        n290 = Equal To 0?(x="aq.mode") -> (x = 0?=w565:bool)
        n291 = Get Date/Time In Seconds() -> (seconds since 1Jan1904=w570:timestamp)
        n292 = for {
          N: w574 -> [w588]
          shift-right: [w608] -> w575
          shift-left: w577 -> [w610]
          shift-right: [w595] -> w573
          shift-left: w576 -> [w609]
          tunnel: w579 -> [w606]
          tunnel: w578 -> [w605]
          tunnel: w569 -> [w604]
          tunnel: w570 -> [w600]
          tunnel: w565 -> [w590]
          shift-right: [w589] -> w564
          shift-left: w568 -> [w591]
          i -> [w585]
          stop <- "abort acq." stop-if-true
          n293 = call "grabimg.vi"("array in"=w604, "error in"=w609, "Hin"=w610) -> ("error out"=w595:errorcluster, "imgdata"=w607:i32[][], "Hout"=w608:u64)  [unwired: 6 in]
          n294 = local read "lower threshold"() -> (w583:i32)
          n295 = Increment(x=w585) -> (x+1=w586:i32)
          "acq. imgs" <- w586
          n296 = Get Date/Time In Seconds() -> (seconds since 1Jan1904=w603:timestamp)
          n297 = case shown="True" w606 {
            tunnel: w607 -> [w632 w635]
            tunnel: w605 -> [_ w634]
            tunnel: [w632 w633] -> w582
            frame False {
            }
            frame True {
              n298 = Subtract(x=w635, y=w634) -> (x-y=w633:dbl[][])
            }
          }
          n299 = Divide(x=w586, y=w588) -> (x/y=→"snap_prog":dbl)
          n300 = Subtract(x=w603, y=w600) -> (x-y=w602:dbl)
          n301 = call "filtr_b.vi"("threshold"=w583, "input array"=w582) -> ("output array"=w581:dbl[][])  [unwired: 9 in]
          n302 = Divide(x=w602, y=w585) -> (x/y=w598:dbl)
          n303 = Multiply(x=w598, y=w588) -> (x*y=w601:dbl)
          n304 = Reciprocal(x=w598) -> (1/x=w597:dbl)
          n305 = case shown="True" "count?" {
            tunnel: w581 -> [w621 w623]
            tunnel: "e-size" -> [_ w625]
            tunnel: w583 -> [_ w624]
            tunnel: [w621 w622] -> w592
            frame False {
            }
            frame True {
              n306 = Array Size(array=w623) -> (size(s)=w627:i32[])
              n307 = call "findr.vi"("thresh"=w624, "esize"=w625, "inp array"=w623) -> ("locs"=w626:i32[][])  [unwired: 8 in]
              n308 = Index Array(array=w627) -> (element #1=w629:i32, element #2=w628:i32)  [unwired: 2 in]
              n309 = call "drawe.vi"("Ysize"=w629, "Xsize"=w628, "pos array"=w626) -> ("img out"=w622:i32[][])  [unwired: 8 in]
            }
          }
          n310 = Add(x=w601, y=w600) -> (x+y=→"ETA":timestamp)
          n311 = local write "cam_fps"(w597) -> ()
          n312 = case shown="True" w590 {
            tunnel: w592 -> [w611 w619]
            tunnel: w585 -> [_ w618]
            tunnel: w591 -> [w613 w617]
            tunnel: [w612 w614] -> w589
            frame False {
              n313 = Add(x=w611, y=w613) -> (x+y=w612:dbl[][])
            }
            frame True {
              n314 = Multiply(x=w617, y=w618) -> (x*y=w620:dbl[][])
              n315 = Increment(x=w618) -> (x+1=w615:i32)
              n316 = Add(x=w619, y=w620) -> (x+y=w616:dbl[][])
              n317 = Divide(x=w616, y=w615) -> (x/y=w614:dbl[][])
            }
          }
          n318 = local write "mainimg"(w581) -> ()
          n319 = Transpose 2D Array(2D array=w581) -> (transposed array=w596:dbl[][])
          n320 = for {
            tunnel: w596 -> [w631] mode=indexing
            tunnel: [w630] -> _ mode=indexing
            n321 = Add Array Elements(numeric array=w631) -> (sum=w630:dbl)
          }
          n322 = local write "sideimg"(w589) -> ()
        }
        n323 = Enqueue Element(queue=w567, element=w564, error in (no error)=w573) -> (error out=w563:errorcluster)  [unwired: 1 in, 2 out]
      }
      frame "suspend" {
        n324 = Dequeue Element(queue=w643) -> ()  [unwired: 2 in, 4 out]
      }
    }
    "cam_error" <- w377
  }
  n325 = while {
    tunnel: w10 -> [w649]
    tunnel: w13 -> [w648]
    tunnel: w3 -> [w647]
    tunnel: w24 -> [w646]
    tunnel: w2 -> [w644]
    tunnel: w11 -> [w645]
    stop <- w650 stop-if-true
    n326 = event shown="[0] Timeout" {
      selector: _ -> [_ _ _ _ _ _ _ _ _ _ _ _ _ _ _ _ _ _ _ _ _ _ _ _ _]
      dyn-events: _ -> [_ _ _ _ _ _ _ _ _ _ _ _ _ _ _ _ _ _ _ _ _ _ _ _ _]
      timeout: _ -> [_ _ _ _ _ _ _ _ _ _ _ _ _ _ _ _ _ _ _ _ _ _ _ _ _]
      tunnel: [_ TRUE _ _ _ _ _ _ _ _ _ _ _ _ _ _ _ _ _ _ _ _ _ _ _] -> w650
      tunnel: w649 -> [_ w663 w666 _ _ _ _ _ w692 w694 _ _ _ _ _ _ _ _ _ _ _ _ _ _ _]
      tunnel: w648 -> [_ w662 _ w670 _ _ _ _ _ _ _ _ _ _ _ _ w725 _ w737 _ _ _ _ _ _]
      tunnel: w647 -> [_ w661 _ _ w676 _ _ _ _ _ _ _ _ w713 _ w717 _ _ _ _ _ _ _ _ _]
      tunnel: w646 -> [_ w660 _ _ _ w682 w688 w689 _ _ _ _ _ _ _ _ _ _ _ _ _ _ _ _ _]
      tunnel: w645 -> [_ w654 _ _ _ _ _ _ _ _ _ _ _ _ _ _ _ _ _ _ _ _ _ _ _]
      tunnel: w644 -> [_ w653 _ _ _ _ _ _ _ _ w696 w698 _ _ w715 _ _ _ _ _ _ _ _ _ _]
      event Timeout {
        n327 = event-data() -> ()  [unwired: 1 in, 1 out]
        n328 = call-poly <vilib>:"Read Delimited Spreadsheet.vi"() -> ("all rows"=w651:string[][])  [unwired: 10 in, 5 out]
        n329 = local write "delay table [fs]"(w651) -> ()
      }
      event "main_close": Value Change {
        w652 = "close" ("element")
        w659 = "release" ("element")
        n330 = event-data() -> ()  [unwired: 1 in, 1 out]
        n331 = Release Queue(queue=w654) -> ()  [unwired: 2 in, 3 out]
        n332 = Enqueue Element(queue=w663, element=w659) -> (queue out=w658:refnum<queue>)  [unwired: 2 in, 2 out]
        n333 = Enqueue Element(queue=w662, element=w659) -> (queue out=w657:refnum<queue>)  [unwired: 2 in, 2 out]
        n334 = Enqueue Element(queue=w661, element=w659) -> (queue out=w656:refnum<queue>)  [unwired: 2 in, 2 out]
        n335 = Enqueue Element(queue=w660, element=w659) -> (queue out=w655:refnum<queue>)  [unwired: 2 in, 2 out]
        n336 = Enqueue Element(queue=w658, element=w652) -> ()  [unwired: 2 in, 3 out]
        n337 = Enqueue Element(queue=w657, element=w652) -> ()  [unwired: 2 in, 3 out]
        n338 = Enqueue Element(queue=w656, element=w652) -> ()  [unwired: 2 in, 3 out]
        n339 = Enqueue Element(queue=w655, element=w652) -> ()  [unwired: 2 in, 3 out]
        n340 = Enqueue Element(queue=w653, element=w652) -> ()  [unwired: 2 in, 3 out]
      }
      event "cam_release", "cam_init": Value Change {
        n341 = event-data() -> ()  [unwired: 1 in, 2 out]
        n342 = Select(t="init" ("name (unnamed)"), s="cam_init", f="release" ("name (unnamed)")) -> (s? t:f=w665:string)
        n343 = Enqueue Element(queue=w666, element=w665) -> ()  [unwired: 2 in, 3 out]
      }
      event "ESP_release", "ESP_init": Value Change {
        n344 = event-data() -> ()  [unwired: 1 in, 2 out]
        n345 = Select(t="init" ("name (unnamed)"), s="ESP_init", f="release" ("name (unnamed)")) -> (s? t:f=w674:string)
        n346 = Enqueue Element(queue=w670, element=w674) -> ()  [unwired: 2 in, 3 out]
      }
      event "manip_init", "manip_release": Value Change {
        n347 = event-data() -> ()  [unwired: 1 in, 2 out]
        n348 = Flush Queue(queue=w676) -> (queue out=w675:refnum<queue>)  [unwired: 1 in, 2 out]
        n349 = Select(t="init" ("name (unnamed)"), s="manip_init", f="release" ("name (unnamed)")) -> (s? t:f=w678:string)
        n350 = Enqueue Element(queue=w675, element=w678) -> ()  [unwired: 2 in, 3 out]
      }
      event "phoib_release", "phoib_init": Value Change {
        n351 = event-data() -> ()  [unwired: 1 in, 2 out]
        n352 = Flush Queue(queue=w682) -> (queue out=w681:refnum<queue>)  [unwired: 1 in, 2 out]
        n353 = Select(t="init" ("name (unnamed)"), s="phoib_init", f="release" ("name (unnamed)")) -> (s? t:f=w684:string)
        n354 = Enqueue Element(queue=w681, element=w684) -> ()  [unwired: 2 in, 3 out]
      }
      event "phoib_standby": Value Change {
        n355 = event-data() -> ()  [unwired: 1 in, 2 out]
        n356 = Enqueue Element(queue=w688, element="standby") -> ()  [unwired: 2 in, 3 out]
      }
      event "phoib_set": Value Change {
        n357 = event-data() -> ()  [unwired: 1 in, 2 out]
        n358 = Enqueue Element(queue=w689, element="set") -> ()  [unwired: 2 in, 3 out]
      }
      event "cam_dark": Value Change {
        n359 = event-data() -> ()  [unwired: 1 in, 2 out]
        n360 = Enqueue Element(queue=w692, element="dark") -> ()  [unwired: 2 in, 3 out]
      }
      event "ROI Left", "ROI Right", "ROI Top", "ROI Bottom", "exposure [ms]", "binning", "gain": Value Change {
        n361 = event-data() -> ()  [unwired: 1 in, 1 out]
        n362 = Enqueue Element(queue=w694, element="set") -> ()  [unwired: 2 in, 3 out]
      }
      event "cam_saveimg": Value Change {
        n363 = event-data() -> ()  [unwired: 1 in, 1 out]
        n364 = Enqueue Element(queue=w696, element="single") -> ()  [unwired: 2 in, 3 out]
      }
      event "delscan_go": Value Change {
        n365 = event-data() -> ()  [unwired: 1 in, 1 out]
        n366 = Enqueue Element(queue=w698, element="GO") -> ()  [unwired: 2 in, 3 out]
      }
      event "Move Abs": Value Change {
        n367 = event-data() -> ()  [unwired: 1 in, 1 out]
      }
      event "ManipRel +", "ManipRel -": Value Change {
        n368 = event-data() -> ()  [unwired: 1 in, 2 out]
        n369 = Negate(x="manip_deltas") -> (-x=w701:dbl[])
        n370 = Select(t="manip_deltas", s="ManipRel +", f=w701) -> (s? t:f=w699:dbl[])
        n371 = Index Array(array=w699) -> (element #1=w705:dbl, element #2=w706:dbl, element #3=w707:dbl, element #4=w708:dbl, element #5=w709:dbl, element #6=w710:dbl)  [unwired: 6 in]
        n372 = Format Into String(format string="%g_%g_%g_%g_%g_%g", w705, w706, w707, w708, w709, w710) -> (resulting string=w712:string)  [unwired: 2 in, 1 out]
        n373 = Concatenate Strings("relative:" ("string"), w712) -> (w703:string)
        n374 = Enqueue Element(queue=w713, element=w703) -> ()  [unwired: 2 in, 3 out]
      }
      event "Optimize": Value Change {
        n375 = event-data() -> ()  [unwired: 1 in, 6 out]
        n376 = Enqueue Element(queue=w715, element="manip") -> ()  [unwired: 2 in, 3 out]
      }
      event "stop manip": Value Change {
        n377 = event-data() -> ()  [unwired: 1 in, 1 out]
        n378 = Enqueue Element(queue=w717, element="stop") -> ()  [unwired: 2 in, 3 out]
      }
      event "ESP_go": Value Change {
        w719 = ":" ("string")
        n379 = event-data() -> ()  [unwired: 1 in, 1 out]
        n380 = local read "ESP Axis"() -> (w718:i32)
        n381 = Number To Decimal String(number=w718) -> (decimal integer string=w721:string)  [unwired: 1 in]
        n382 = Number To Fractional String(number="ESP_dest") -> (F-format string=w720:string)  [unwired: 3 in]
        n383 = Concatenate Strings("abs:" ("string"), w721, w719, w720, w719) -> (w724:string)
        n384 = Enqueue Element(queue=w725, element=w724) -> ()  [unwired: 2 in, 3 out]
      }
      event "ESP_set_t0": Value Change {
        n385 = event-data() -> ()  [unwired: 1 in, 1 out]
        n386 = Current VI's Path() -> (path=w731:path)
        n387 = Strip Path(path=w731) -> (stripped path=w727:path)  [unwired: 1 out]
        n388 = Strip Path(path=w727) -> (stripped path=w726:path)  [unwired: 1 out]
        n389 = local read "ESP_pos"() -> (w729:dbl)
        "ESP_t0" <- w729
        n390 = Number To Fractional String(number=w729) -> (F-format string=w728:string)  [unwired: 3 in]
        n391 = Build Path(base path=w726, name or relative path="t0.txt") -> (appended path=w730:path)
        n392 = Write to Text File(file (use dialog)=w730, text=w728) -> ()  [unwired: 2 in, 3 out]
      }
      event "ESP_+", "ESP_-": Value Change {
        n393 = event-data() -> ()  [unwired: 1 in, 6 out]
        n394 = Negate(x="ESP_delta") -> (-x=w740:dbl)
        n395 = Select(t="ESP_delta", s="ESP_+", f=w740) -> (s? t:f=w738:dbl)
        n396 = Number To Decimal String(number="ESP Axis") -> (decimal integer string=w735:string)  [unwired: 1 in]
        n397 = Number To Fractional String(number=w738) -> (F-format string=w733:string)  [unwired: 3 in]
        n398 = Concatenate Strings("rel:" ("string"), w735, ":" ("string"), w733) -> (w743:string)
        n399 = Enqueue Element(queue=w737, element=w743) -> ()  [unwired: 2 in, 3 out]
      }
      event "ESP_dest": Value Change {
        n400 = event-data() -> ()  [unwired: 1 in, 6 out]
        n401 = local read "ESP_dest"() -> (w747:dbl)
        n402 = local read "ESP_t0"() -> (w746:dbl)
        n403 = call "mm2time.vi"("fs?"=TRUE ("fs[1]/ps[0]"), "Offset (mm)"=w746, "distance (mm)"=w747) -> ("time in fs/ps seconds"=w744:dbl)
        n404 = local write "ESP_dest_t"(w744) -> ()
      }
      event "ESP_dest_t": Value Change {
        n405 = event-data() -> ()  [unwired: 1 in, 1 out]
        n406 = local read "ESP_t0"() -> (w750:dbl)
        n407 = call "time2mm.vi"("fs[1]/ps[0]"=TRUE, "Offset (mm)"=w750, "time"="ESP_dest_t") -> ("position (mm)"=w748:dbl)
        n408 = local write "ESP_dest"(w748) -> ()
      }
      event "load delay table": Value Change {
        n409 = event-data() -> ()  [unwired: 1 in, 6 out]
        n410 = call-poly <vilib>:"Read Delimited Spreadsheet.vi"() -> ("all rows"=w753:string[][])  [unwired: 10 in, 5 out]
        n411 = local read "binning"() -> (w760:u16)
        n412 = local write "delay table [fs]"(w753) -> ()
        n413 = local read "delscan_iters"() -> (w754:u32)
        n414 = local read "time / step"() -> (w763:dbl)
        n415 = Array Size(array=w753) -> (size(s)=w764:i32[])
        n416 = Index Array(array=dbl[] [8.79, 2.2, 0.553, 0.138], index=w760) -> (element=w758:dbl)
        n417 = Index Array(array=w764) -> (element #1=w752:i32)  [unwired: 2 in, 1 out]
        n418 = Multiply(x=w754, y=w752) -> (x*y=w757:u32)
        n419 = Multiply(x=w752, y=w758) -> (x*y=w759:dbl)
        n420 = Multiply(x=w757, y=w763) -> (x*y=w762:dbl)
        n421 = Increment(x=w757) -> (x+1=w756:u32)
        n422 = Multiply(x=w756, y=w758) -> (x*y=w755:dbl)
        n423 = local write "delaypoints"(w752) -> ()
        n424 = local write "total steps"(w757) -> ()
        n425 = local write "duration [HH:MM:SS]"(w762) -> ()
        n426 = local write "RAM [MB]"(w759) -> ()
        n427 = local write "disk [MB]"(w755) -> ()
      }
      event "delay table [fs]", "delscan_iters": Value Change {
        n428 = event-data() -> ()  [unwired: 1 in, 6 out]
        n429 = local read "binning"() -> (w773:u16)
        n430 = local read "delay table [fs]"() -> (w777:string[][])
        n431 = local read "delscan_iters"() -> (w767:u32)
        n432 = local read "time / step"() -> (w775:dbl)
        n433 = Array Size(array=w777) -> (size(s)=w776:i32[])
        n434 = Index Array(array=dbl[] [8.79, 2.2, 0.553, 0.138], index=w773) -> (element=w771:dbl)
        n435 = Index Array(array=w776) -> (element #1=w765:i32)  [unwired: 2 in, 1 out]
        n436 = Multiply(x=w767, y=w765) -> (x*y=w770:u32)
        n437 = Multiply(x=w765, y=w771) -> (x*y=w772:dbl)
        n438 = Multiply(x=w770, y=w775) -> (x*y=w774:dbl)
        n439 = Increment(x=w770) -> (x+1=w769:u32)
        n440 = Multiply(x=w769, y=w771) -> (x*y=w768:dbl)
        n441 = local write "delaypoints"(w765) -> ()
        n442 = local write "total steps"(w770) -> ()
        n443 = local write "duration [HH:MM:SS]"(w774) -> ()
        n444 = local write "RAM [MB]"(w772) -> ()
        n445 = local write "disk [MB]"(w768) -> ()
      }
      event "generate delay table": Value Change {
        n446 = event-data() -> ()  [unwired: 1 in, 1 out]
        n447 = call "getdelaypoints.vi"("delscan_stepsize"="delscan_stepsize", "delscan_end"="delscan_end", "delscan_start"="delscan_start") -> ("delaypoints"=w793:dbl[])
        n448 = Number To Fractional String(number=w793) -> (F-format string=w792:string[])  [unwired: 3 in]
        n449 = Build Array(w792) -> (w791:string[][])
        n450 = Transpose 2D Array(2D array=w791) -> (transposed array=w778:string[][])
        n451 = local write "delay table [fs]"(w778) -> ()
        n452 = local read "binning"() -> (w787:u16)
        n453 = local read "delscan_iters"() -> (w781:u32)
        n454 = local read "time / step"() -> (w789:dbl)
        n455 = Array Size(array=w778) -> (size(s)=w790:i32[])
        n456 = Index Array(array=dbl[] [8.79, 2.2, 0.553, 0.138], index=w787) -> (element=w785:dbl)
        n457 = Index Array(array=w790) -> (element #1=w779:i32)  [unwired: 2 in, 1 out]
        n458 = Multiply(x=w781, y=w779) -> (x*y=w784:u32)
        n459 = Multiply(x=w779, y=w785) -> (x*y=w786:dbl)
        n460 = Multiply(x=w784, y=w789) -> (x*y=w788:dbl)
        n461 = Increment(x=w784) -> (x+1=w783:u32)
        n462 = Multiply(x=w783, y=w785) -> (x*y=w782:dbl)
        n463 = local write "delaypoints"(w779) -> ()
        n464 = local write "total steps"(w784) -> ()
        n465 = local write "duration [HH:MM:SS]"(w788) -> ()
        n466 = local write "RAM [MB]"(w786) -> ()
        n467 = local write "disk [MB]"(w782) -> ()
      }
      event "mainimg": Cursor Release {
        n468 = event-data() -> ()  [unwired: 1 in, 1 out]
      }
    }
  }
  n469 = while {
    tunnel: w13 -> [w805]
    shift-right: [w803] -> _
    shift-left: _ -> [w801]
    shift-right: [w802] -> _
    shift-left: _ -> [w800]
    shift-right: [w798] -> _
    shift-left: 0 -> [w799]
    tunnel: w2 -> [w797]
    stop <- w804 stop-if-true
    # "ESP"
    n470 = Preview Queue Element(queue=w805, timeout in ms (-1)=w799) -> (queue out=w808:refnum<queue>, element=w809:string)  [unwired: 1 in, 2 out]
    n471 = Match Pattern(string=w809, regular expression=":") -> (before substring=w807:string, after substring=w806:string)  [unwired: 1 in, 2 out]
    n472 = case shown="\"idle\", Default" w807 {
      tunnel: w808 -> [_ w820 w838 w872 w873 w880 w885]
      tunnel: w806 -> [_ w825 w845 _ _ _ _]
      tunnel: [_ _ _ _ _ TRUE _] -> w804
      tunnel: [w812 w827 w839 w870 refnum<visa-resource-name> refnum ("VISA resource name out") w877 w884] -> w803
      tunnel: [w811 w828 w837 w869 w875 w878 w883] -> w802
      tunnel: w801 -> [w816 w830 w843 w870 w876 w877 _]
      tunnel: w800 -> [w815 w829 w844 w869 _ w878 _]
      tunnel: [_ _ _ -1 _ _ _] -> w798
      tunnel: w797 -> [_ _ w836 _ _ _ _]
      frame "idle", Default {
        n473 = local read "ESP Axis"() -> (w813:i32)
        n474 = local read "ESP_t0"() -> (w819:dbl)
        n475 = call "Read Actual Position.vi"("error in (no error)"=w815, "Axis (1)"=w813, "VISA resource name"=w816) -> ("error out"=w811:errorcluster, "Position (units)"=w814:dbl, "VISA resource name out"=w812:refnum<visa-resource-name>)  [unwired: 2 in]
        "ESP_pos" <- w814
        n476 = call "mm2time.vi"("fs?"=TRUE, "Offset (mm)"=w819, "distance (mm)"=w814) -> ("time in fs/ps seconds"=→"ESP_delay":dbl)
      }
      frame "rel" {
        n477 = Match Pattern(string=w825, regular expression=":") -> (before substring=w824:string, after substring=w823:string)  [unwired: 1 in, 2 out]
        n478 = Dequeue Element(queue=w820) -> ()  [unwired: 2 in, 4 out]
        n479 = Decimal String To Number(string=w824) -> (number=w822:i32)  [unwired: 2 in, 1 out]
        n480 = Fract/Exp String To Number(string=w823) -> (number=w821:dbl)  [unwired: 3 in, 1 out]
        n481 = call "Move Relative.vi"("error in (no error)"=w829, "Position (0 units)"=w821, "Axis (1)"=w822, "VISA resource name"=w830) -> ("error out"=w828:errorcluster, "VISA resource name out"=w827:refnum<visa-resource-name>)  [unwired: 2 in]
      }
      frame "abs" {
        n482 = Dequeue Element(queue=w838) -> ()  [unwired: 2 in, 4 out]
        n483 = Match Pattern(string=w845, regular expression=":") -> (before substring=w846:string, after substring=w834:string)  [unwired: 1 in, 2 out]
        n484 = Match Pattern(string=w834, regular expression=":") -> (before substring=w833:string, after substring=w832:string)  [unwired: 1 in, 2 out]
        n485 = Decimal String To Number(string=w846) -> (number=w842:i32)  [unwired: 2 in, 1 out]
        n486 = Fract/Exp String To Number(string=w833) -> (number=w831:dbl)  [unwired: 3 in, 1 out]
        n487 = call "Move Absolute.vi"("error in (no error)"=w844, "Position (0 units)"=w831, "Axis (1)"=w842, "VISA resource name"=w843) -> ("error out"=w840:errorcluster, "VISA resource name out"=w841:refnum<visa-resource-name>)  [unwired: 2 in]
        n488 = case shown="\"wait\"" w832 {
          tunnel: w842 -> [_ w854]
          tunnel: w841 -> [w849 w859]
          tunnel: w840 -> [w848 w858]
          tunnel: [w849 w851] -> w839
          tunnel: [w848 w857] -> w837
          tunnel: w836 -> [_ w856]
          frame "", Default {
          }
          frame "wait" {
            n489 = while {
              tunnel: w854 -> [w868]
              shift-right: [w865] -> w853
              shift-left: w859 -> [w867]
              shift-right: [w864] -> w852
              shift-left: w858 -> [w866]
              stop <- w863 stop-if-true
              n490 = call "Get Axis Motion Status.vi"("error in (no error)"=w866, "Axis (1)"=w868, "VISA resource name"=w867) -> ("error out"=w864:errorcluster, "Motion Done"=w863:bool, "VISA resource name out"=w865:refnum<visa-resource-name>)  [unwired: 2 in]
            }
            n491 = flat-sequence {
              tunnel: w853 -> [w862]
              tunnel: w852 -> [w861]
              tunnel: [w862] -> w851
              tunnel: [w861] -> w850
              frame #0 {
                n492 = Wait (ms)(milliseconds to wait=u32 1000) -> ()  [unwired: 1 out]
              }
            }
            n493 = Enqueue Element(queue=w856, element="done", error in (no error)=w850) -> (error out=w857:errorcluster)  [unwired: 1 in, 2 out]
          }
        }
      }
      frame "suspend" {
        n494 = Dequeue Element(queue=w872) -> ()  [unwired: 2 in, 4 out]
      }
      frame "release" {
        n495 = Dequeue Element(queue=w873) -> ()  [unwired: 2 in, 4 out]
        n496 = call "Close.vi"("VISA resource name"=w876) -> ("error out"=w875:errorcluster)  [unwired: 10 in]
      }
      frame "close" {
        n497 = Release Queue(queue=w880) -> ()  [unwired: 2 in, 3 out]
      }
      frame "init" {
        n498 = Dequeue Element(queue=w885) -> ()  [unwired: 2 in, 4 out]
        n499 = flat-sequence {
          tunnel: [w888] -> w882
          tunnel: [w887] -> w881
          tunnel: [w892] -> w883
          tunnel: [w893] -> w884
          tunnel: w882 -> [w893]
          tunnel: w881 -> [w892]
          frame #0 {
            n500 = local write "ESP_con?"(FALSE ("ESP_con?")) -> ()
          }
          frame #1 {
            n501 = call "Initialize.vi"("VISA resource name"="ESP301 VISA", "Serial Link (RS232)"=enum16{"RS232", "USB"}."USB") -> ("VISA resource name out"=w888:refnum<visa-resource-name>, "error out"=w887:errorcluster)  [unwired: 7 in]
          }
          frame #2 {
            n502 = local write "ESP_con?"(TRUE ("ESP_con?")) -> ()
          }
        }
      }
    }
    "error out" <- w802
  }
  n503 = while {
    tunnel: w3 -> [w902]
    shift-right: [w900] -> _
    shift-left: _ -> [w898]
    shift-right: [w899] -> _
    shift-left: _ -> [w897]
    shift-right: [w895] -> _
    shift-left: 0 -> [w896]
    tunnel: w2 -> [w894]
    stop <- w901 stop-if-true
    # "manip"
    n504 = Preview Queue Element(queue=w902, timeout in ms (-1)=w896) -> (queue out=w905:refnum<queue>, element=w906:string)  [unwired: 1 in, 2 out]
    n505 = Match Pattern(string=w906, regular expression=":") -> (before substring=w904:string, after substring=w903:string)  [unwired: 1 in, 2 out]
    n506 = case shown="\"init\"" w904 {
      tunnel: w905 -> [_ w918 w945 w972 w976 w985 w990]
      tunnel: w903 -> [_ _ w932 _ _ _ _]
      tunnel: [_ _ _ _ _ TRUE _] -> w901
      tunnel: [w912 w920 w924 w974 refnum<k5> refnum ("gateway_connection out") w983 w989] -> w900
      tunnel: [w911 w919 w926 w973 w978 w982 w988] -> w899
      tunnel: w898 -> [w914 w922 w948 w974 w980 w983 _]
      tunnel: w897 -> [w913 w921 w947 w973 _ w982 _]
      tunnel: [_ _ _ -1 _ _ _] -> w895
      tunnel: w894 -> [_ _ w923 _ _ _ _]
      frame "idle", Default {
        n507 = call "sp_manip_get_axis_status.vi"("error in"=w913, "gateway_connection"=w914) -> ("error out"=w911:errorcluster, "axis_out"=w910:T7, "gateway_connection out"=w912:refnum<k5>)  [unwired: 5 in, 2 out]
        n508 = for {
          tunnel: w910 -> [w917] mode=indexing
          tunnel: [w916] -> w909 mode=indexing
          tunnel: [w915] -> w908 mode=indexing
          n509 = Unbundle By Name(w917) -> ("Axis_Position"=w916:dbl, "moving"=w915:bool)
        }
        "moving?" <- w908
        n510 = local write "pos"(w909) -> ()
      }
      frame "stop" {
        n511 = Dequeue Element(queue=w918) -> ()  [unwired: 2 in, 4 out]
        n512 = call "sp_manip_abort.vi"("error in"=w921, "gateway_connection"=w922) -> ("error out"=w919:errorcluster, "gateway_connection out"=w920:refnum<k5>)  [unwired: 6 in, 2 out]
      }
      frame "relative" {
        n513 = Dequeue Element(queue=w945) -> ()  [unwired: 2 in, 4 out]
        n514 = Match Pattern(string=w932, regular expression=":") -> (before substring=w931:string, after substring=w930:string)  [unwired: 1 in, 2 out]
        n515 = Equal?(x=w930, y="wait") -> (x = y?=w928:bool)
        n516 = call "sp_manip_get_axis_status.vi"("error in"=w947, "gateway_connection"=w948) -> ("error out"=w950:errorcluster, "axis_out"=w937:T7, "gateway_connection out"=w949:refnum<k5>)  [unwired: 5 in, 2 out]
        n517 = Scan From String(format string="%g_%g_%g_%g_%g_%g", input string=w931) -> (output 1=w944:dbl, output 2=w943:dbl, output 3=w942:dbl, output 4=w941:dbl, output 5=w940:dbl, output 6=w939:dbl)  [unwired: 8 in, 3 out]
        n518 = for {
          tunnel: w937 -> [w971] mode=indexing
          tunnel: [w970] -> w935 mode=indexing
          tunnel: [w969] -> w936 mode=indexing
          n519 = Unbundle By Name(w971) -> ("Axis_Name"=w970:string, "Axis_Position"=w969:dbl)
        }
        n520 = Build Array(w944, w943, w942, w941, w940, w939) -> (w938:dbl[])
        n521 = Add(x=w936, y=w938) -> (x+y=w934:dbl[])
        n522 = call "sp_manip_start_move.vi"("error in"=w950, "target positions"=w934, "axis names"=w935, "gateway_connection"=w949) -> ("error out"=w927:errorcluster, "gateway_connection out"=w925:refnum<k5>)  [unwired: 4 in, 2 out]
        n523 = case shown="True" w928 {
          tunnel: w927 -> [w951 w958]
          tunnel: [w951 w954] -> w926
          tunnel: w925 -> [w952 w959]
          tunnel: [w952 w957] -> w924
          tunnel: w923 -> [_ w953]
          frame False {
          }
          frame True {
            n524 = while {
              tunnel: w959 -> [w963]
              tunnel: w958 -> [w962]
              tunnel: [w961] -> w957
              tunnel: [w960] -> w955
              stop <- w964 continue-if-true
              n525 = call "sp_manip_get_axis_status.vi"("error in"=w962, "gateway_connection"=w963) -> ("error out"=w960:errorcluster, "axis_out"=w966:T7, "gateway_connection out"=w961:refnum<k5>)  [unwired: 5 in, 2 out]
              n526 = for {
                tunnel: w966 -> [w968] mode=indexing
                tunnel: [w967] -> w965 mode=indexing
                n527 = Unbundle By Name(w968) -> ("moving"=w967:bool)
              }
              n528 = Or Array Elements(Boolean array=w965) -> (logical OR=w964:bool)
            }
            n529 = Enqueue Element(queue=w953, element="done", error in (no error)=w955) -> (error out=w954:errorcluster)  [unwired: 1 in, 2 out]
          }
        }
      }
      frame "suspend" {
        n530 = Dequeue Element(queue=w972) -> ()  [unwired: 2 in, 4 out]
      }
      frame "release" {
        n531 = Dequeue Element(queue=w976) -> ()  [unwired: 2 in, 4 out]
        n532 = call "sp_manip_disconnect.vi"("gateway_connection"=w980) -> ("error out"=w979:errorcluster, "gateway_connection_out"=w981:refnum<k5>)  [unwired: 7 in, 2 out]
        n533 = call "tcp_gateway_close_connection.vi"("error in"=w979, "server_connection"=w981) -> ("error out"=w978:errorcluster)  [unwired: 5 in]
      }
      frame "close" {
        n534 = Release Queue(queue=w985) -> ()  [unwired: 2 in, 3 out]
      }
      frame "init" {
        n535 = Dequeue Element(queue=w990) -> ()  [unwired: 2 in, 4 out]
        n536 = flat-sequence {
          tunnel: [w993] -> w987
          tunnel: [w992] -> w986
          tunnel: [w1003] -> w988
          tunnel: [w1004] -> w989
          tunnel: w987 -> [w1004]
          tunnel: w986 -> [w1003]
          frame #0 {
            n537 = local write "manip_con?"(FALSE ("manip_con?")) -> ()
          }
          frame #1 {
            n538 = call "tcp_gateway_open_connection.vi"() -> ("gateway_connection"=w996:refnum<k5>, "error out"=w995:errorcluster)  [unwired: 5 in, 3 out]
            n539 = call "sp_manip_connect.vi"("error in"=w995, "gateway_connection"=w996) -> ("error out"=w992:errorcluster, "axis_out"=w994:T7, "gateway_connection out"=w993:refnum<k5>)  [unwired: 5 in, 2 out]
            n540 = for {
              tunnel: w994 -> [w1001] mode=indexing
              tunnel: [w1000] -> w997 mode=indexing
              tunnel: [w999] -> w998 mode=indexing
              n541 = Unbundle By Name(w1001) -> ("Axis_Name"=w1000:string, "Axis_Position"=w999:dbl)
            }
            "axis" <- w997
            "pos" <- w998
            n542 = local write "dest"(w998) -> ()
          }
          frame #2 {
            n543 = local write "manip_con?"(TRUE ("manip_con?")) -> ()
          }
        }
      }
    }
    "error out 2" <- w899
  }
  n544 = while {
    tunnel: w24 -> [w1015]
    shift-right: [w1012] -> _
    shift-left: 0 -> [w1013]
    shift-right: [w1011] -> _
    shift-left: _ -> [w1010]
    shift-right: [w1009] -> _
    shift-left: _ -> [w1008]
    shift-right: [w1007] -> _
    shift-left: u32 0 ("pHandle") -> [w1006]
    tunnel: string[] ["Kinetic Energy", "Pass Energy", "Coil Current", "Work Function", "Detector Voltage", "Screen Voltage", "Conversion Voltage", "Focus Displacement 1", "Focus Displacement 2"] -> [w1005]
    stop <- w1014 stop-if-true
    # "phoib"
    n545 = Preview Queue Element(queue=w1015, timeout in ms (-1)=w1013) -> (queue out=w1018:refnum<queue>, element=w1019:string)  [unwired: 1 in, 2 out]
    n546 = Match Pattern(string=w1019, regular expression=":") -> (before substring=w1017:string, after substring=w1016:string)  [unwired: 1 in, 2 out]
    n547 = case shown="\"standby\"" w1017 {
      tunnel: w1018 -> [_ w1072 w1088 w1104 w1118 w1122 w1128]
      tunnel: w1016 -> [_ _ _ _ _ _ _]
      tunnel: [_ _ _ _ TRUE _ _] -> w1014
      tunnel: [_ _ _ _ _ -1 _] -> w1012
      tunnel: [w1029 w1074 w1091 w1102 w1116 w1121 w1125] -> w1011
      tunnel: w1010 -> [w1040 w1063 w1093 w1103 w1116 w1121 _]
      tunnel: [w1028 w1073 w1090 w1101 w1114 w1119 w1124] -> w1009
      tunnel: w1008 -> [w1038 w1062 w1092 _ w1114 w1119 _]
      tunnel: [w1026 w1060 w1089 w1100 w1115 w1120 w1127] -> w1007
      tunnel: w1006 -> [w1026 w1060 w1089 w1099 w1115 w1120 _]
      tunnel: w1005 -> [w1027 w1053 _ _ _ _ _]
      frame "idle", Default {
        n548 = call "SL2_AD_DLL_Phoibos_GetDeviceState.vi"("dll_path"=w1040, "pHandle_in"=w1026, "dev_type"=DEF_dev_type."devA (analyzer)", "error in"=w1038) -> ("path out"=w1025:path, "state"=→"state":T3, "error out"=w1024:errorcluster)  [unwired: 2 in]
        n549 = for {
          tunnel: w1026 -> [w1047]
          tunnel: w1027 -> [w1045] mode=indexing
          tunnel: [w1044] -> w1037 mode=indexing
          tunnel: [w1043] -> w1029
          shift-right: [w1042] -> w1028
          shift-left: w1024 -> [w1046]
          tunnel: w1025 -> [w1041]
          n550 = call "SL2_AD_DLL_Phoibos_GetVoltage.vi"("error in"=w1046, "voltage_name"=w1045, "pHandle"=w1047, "dll path in"=w1041) -> ("error out"=w1042:errorcluster, "value"=w1044:dbl, "dll path out"=w1043:path)  [unwired: 3 in]
        }
        n551 = Index Array(array=w1037) -> (element #1=→"phoib_I_1":dbl, element #2=→"phoib_I_2":dbl, element #3=→"phoib_I_3":dbl, element #4=→"phoib_I_4":dbl, element #5=→"phoib_I_5":dbl, element #6=→"phoib_I_6":dbl, element #7=→"phoib_I_7":dbl, element #8=→"phoib_I_8":dbl, element #9=→"phoib_I_9":dbl)  [unwired: 9 in]
      }
      frame "set" {
        n552 = Dequeue Element(queue=w1072) -> ()  [unwired: 2 in, 4 out]
        n553 = Multiply(x="VoltageRange", y=13) -> (x*y=w1069:i32)
        n554 = Add(x="Mode", y=w1069) -> (x+y=w1066:i32)
        n555 = Index Array(array=u32[] [251749632, 251749633, 251749634, 251749635, 251749636, 251749637, 251749638, 251749639, 251749640, 251749641, 251749642, 251749643, 251749644, 251749645, 251749646, 251749647, 251749648, 251749649, 251749650, 251749651, 251749652, 251749653, 251749654, 251749655, 251749656, 251749657, 251749658, 251749659, 251749660, 251749661, 251749662, 251749663, 251749664, 251749665, 251749666, 251749667, 251749668, 251749669, 251749670, 251749671, 251749672, 251749673, 251749674, 251749675, 251749676, 251749677, 251749678, 251749679, 251749680, 251749681, 251749682, 251749683, 251749684, 251749685, 251749686, 251749687, 251749688, 251749689, 251749690, 251749691, 251749692, 251749693, 251749694, 251749695, 251749696] ("modeIDs"), index=w1066) -> (element=w1064:u32)
        n556 = Build Array("phoib_I_1s", "phoib_I_2s", "phoib_I_3s", "phoib_I_4s", "phoib_I_5s", "phoib_I_6s", "phoib_I_7s", "phoib_I_8s", "phoib_I_9s") -> (w1052:dbl[])
        n557 = call "SL2_AD_DLL_Phoibos_SetDeviceMode.vi"("pHandle"=w1060, "error in"=w1062, "value"=w1064, "dev_type"=DEF_dev_type."devA (analyzer)", "dll path in"=w1063) -> ("error out"=w1051:errorcluster, "dll path out"=w1061:path)  [unwired: 4 in]
        n558 = for {
          tunnel: w1060 -> [w1080]
          shift-right: [w1087] -> w1074
          shift-left: w1061 -> [w1084]
          tunnel: w1053 -> [w1079] mode=indexing
          tunnel: w1052 -> [w1078] mode=indexing
          shift-right: [w1086] -> w1073
          shift-left: w1051 -> [w1082]
          n559 = call "SL2_AD_DLL_Phoibos_GetVoltageRange.vi"("error in"=w1082, "voltage_name"=w1079, "pHandle"=w1080, "dll path in"=w1084) -> ("error out"=w1081:errorcluster, "min"=w1076:dbl, "max"=w1077:dbl, "dll path out"=w1083:path)  [unwired: 2 in]
          n560 = In Range and Coerce(upper limit=w1077, x=w1078, lower limit=w1076) -> (coerced(x)=w1075:dbl)  [unwired: 1 out]
          n561 = call "SL2_AD_DLL_Phoibos_SetVoltage.vi"("commit"=TRUE, "pHandle"=w1080, "error in"=w1081, "value"=w1075, "voltageName"=w1079, "dll path in"=w1083) -> ("error out"=w1086:errorcluster, "dll path out"=w1087:path)  [unwired: 3 in]
        }
      }
      frame "standby" {
        w1094 = T3 0 items=["Off"=-1, "Standby"=0, "On"=1] ("state")
        n562 = Dequeue Element(queue=w1088) -> ()  [unwired: 2 in, 4 out]
        n563 = call "SL2_AD_DLL_Phoibos_SetDeviceState.vi"("pHandle_in"=w1089, "error in"=w1092, "state"=w1094, "dev_type"=DEF_dev_type."devA (analyzer)", "dll_path"=w1093) -> ("error out"=w1090:errorcluster, "path out"=w1091:path)  [unwired: 2 in]
      }
      frame "release" {
        n564 = Dequeue Element(queue=w1104) -> ()  [unwired: 2 in, 4 out]
        n565 = flat-sequence {
          tunnel: w1103 -> [w1105]
          tunnel: w1099 -> [w1106]
          tunnel: [w1109] -> w1098
          tunnel: [w1108] -> w1097
          tunnel: [u32 0] -> w1096
          tunnel: [w1111] -> w1100
          tunnel: [w1112] -> w1101
          tunnel: [w1113] -> w1102
          tunnel: w1098 -> [w1113]
          tunnel: w1097 -> [w1112]
          tunnel: w1096 -> [w1111]
          frame #0 {
            n566 = call "SL2_AD_DLL_Phoibos_Shutdown.vi"("pHandle"=w1106, "dll path in"=w1105) -> ("error out"=w1108:errorcluster, "dll path out"=w1109:path)  [unwired: 4 in]
          }
          frame #1 {
            n567 = local write "phoib_con?"(FALSE ("phoib_con?")) -> ()
          }
        }
      }
      frame "close" {
        n568 = Release Queue(queue=w1118) -> ()  [unwired: 2 in, 3 out]
      }
      frame "suspend" {
        n569 = Dequeue Element(queue=w1122) -> ()  [unwired: 2 in, 4 out]
      }
      frame "init" {
        n570 = Dequeue Element(queue=w1128) -> ()  [unwired: 2 in, 4 out]
        n571 = flat-sequence {
          tunnel: [w1135] -> w1126
          tunnel: [w1131] -> w1125
          tunnel: [w1130] -> w1124
          tunnel: [w1143] -> w1127
          tunnel: w1126 -> [w1143]
          frame #0 {
            n572 = local write "phoib_con?"(FALSE ("phoib_con?")) -> ()
          }
          frame #1 {
            w1134 = DEF_dev_type."devA (analyzer)" ("dev_type")
            n573 = call "GetSL2AD_VI_dllPath.vi"() -> ("error"=w1138:errorcluster, "Path"=w1139:path)  [unwired: 9 in, 1 out]
            n574 = call "SL2_AD_DLL_List_Devices.vi"("error in"=w1138, "dev_type"=w1134, "dll path in"=w1139) -> ("error out"=w1132:errorcluster, "devices"=w1141:string[], "dll path out"=w1133:path)  [unwired: 2 in]
            n575 = Index Array(array=w1141) -> (element=w1140:string)  [unwired: 1 in]
            n576 = call "SL2_AD_DLL_Phoibos_Initialize.vi"("error in"=w1132, "analyzerId"=w1140, "dll_path"=w1133) -> ("error out"=w1136:errorcluster, "pHandle"=w1135:u32, "path out"=w1137:path)  [unwired: 2 in]
            n577 = call "SL2_AD_DLL_Phoibos_ListDeviceModes.vi"("dll path in"=w1137, "dev_type"=w1134, "pHandle"=w1135, "error in"=w1136) -> ("dll path out"=w1131:path, "error out"=w1130:errorcluster)  [unwired: 1 in, 2 out]
          }
          frame #2 {
            n578 = local write "phoib_con?"(TRUE ("phoib_con?")) -> ()
          }
        }
      }
    }
    "phoib_error" <- w1009
  }
